vi "TestExecutive V3.vi"() -> ()   [LabVIEW 2025]
uses:
  controls/TestDefinition.ctl
  controls/SingleTest.ctl
  controls/TestType.ctl
  controls/Diode Test Options.ctl
  controls/HTR Test Options.ctl
  controls/TED4015 Status.ctl
  <vilib>/Utility/error.llb/DialogType.ctl
  <vilib>/addons/_JKI Toolkits/State Machine/_JKI_lib_State_Machine.llb/Select State(s)_err__jki_lib_state_machine.vi
  <vilib>/addons/_JKI Toolkits/State Machine/_JKI_lib_State_Machine.llb/Periodic Trigger__ogtk__JKI-SM__jki_lib_state_machine.vi
  subVIs/Globals.vi
panel:
  in  "Exit":bool
  out "Camera":string="HD Pro Webcam C920"
  out "TopFolderPath":path=path "D:/LTM Tests/November/Diode_check_25-11-13_18-53-57"
  out "TopFolderPrefix":string="Diode_check_25-11-13_18-53-57"
  out "Status":string="Waiting for Rising trigger. Target = -50.000000"
  in  "Main Tabs":T1(tab)=enum."Operating"
  in  "Cycles To Run":i32=1 min=1 max=200
  in  "Next1":bool
  in  "Loggers Directory":path=path "D:/LTM Tests/November"
  in  "Test Name":string="ChamberInstall_Pre-Test_Step47"
  in  "FFMPEG exe":path=path "C:/Program Files/FFMpeg/bin/ffmpeg.exe"
  in  "Path to Actuation Script":path=path "C:/Users/dpl/Documents/ob-egse/src/main.py"
  in  "StartCycle":i32
  in  "Tab Control":T2(tab)=enum."PSUs"
  in  "TVC_Temperatures":waveform(dbl)[](array[waveform])=[{"t0"=timestamp(3845904937.0241175 s since 1904-01-01), "dt"=1.0, "Y"=[-80.0], "attributes"=variant("NI_ChannelName"=variant(string "3A"))}, {"t0"=timestamp(3845904937.0241175 s since 1904-01-01), "dt"=1.0, "Y"=[0.1969585335155295], "attributes"=variant("NI_ChannelName"=variant(string "3B"))}, {"t0"=timestamp(3845904937.0241175 s since 1904-01-01), "dt"=1.0, "Y"=[0.2898606356704896], "attributes"=variant("NI_ChannelName"=variant(string "3C"))}, {"t0"=timestamp(3845904937.0241175 s since 1904-01-01), "dt"=1.0, "Y"=[0.3274623555028864], "attributes"=variant("NI_ChannelName"=variant(string "3D"))}, {"t0"=timestamp(3845904937.0241175 s since 1904-01-01), "dt"=1.0, "Y"=[0.3794250746071903], "attributes"=variant("NI_ChannelName"=variant(string "4A"))}, {"t0"=timestamp(3845904937.0241175 s since 1904-01-01), "dt"=1.0, "Y"=[0.7650917242886434], "attributes"=variant("NI_ChannelName"=variant(string "4B"))}, {"t0"=timestamp(3845904937.0241175 s since 1904-01-01), "dt"=1.0, "Y"=[0.4416685188806395], "attributes"=variant("NI_ChannelName"=variant(string "4C"))}, {"t0"=timestamp(3845904937.0241175 s since 1904-01-01), "dt"=1.0, "Y"=[0.7497510727682433], "attributes"=variant("NI_ChannelName"=variant(string "4D"))}, {"t0"=timestamp(3845904937.0241175 s since 1904-01-01), "dt"=1.0, "Y"=[0.8015992709050663], "attributes"=variant("NI_ChannelName"=variant(string "Target"))}]
  out "ChannelNames":string[](array[string])=["3A", "3B", "3C", "3D", "4A", "4B", "4C", "4D", "Target"]
  in  "ControlChannel":u16(ring) items=["3A", "3B", "3C", "3D", "4A", "4B", "4C", "4D", "Target"]
  in  "TLUP_Temperatures":waveform(dbl)[](array[waveform])=[{"t0"=timestamp(3820413812.102944 s since 1904-01-01), "dt"=1.0, "Y"=[23.56152], "attributes"=variant("NI_ChannelName"=variant(string "TLUP_0"))}, {"t0"=timestamp(3820413812.102944 s since 1904-01-01), "dt"=1.0, "Y"=[-999.0], "attributes"=variant("NI_ChannelName"=variant(string "TLUP_1"))}, {"t0"=timestamp(3820413812.102944 s since 1904-01-01), "dt"=1.0, "Y"=[-999.0], "attributes"=variant("NI_ChannelName"=variant(string "TLUP_2"))}, {"t0"=timestamp(3820413812.102944 s since 1904-01-01), "dt"=1.0, "Y"=[-999.0], "attributes"=variant("NI_ChannelName"=variant(string "TLUP_3"))}, {"t0"=timestamp(3820413812.102944 s since 1904-01-01), "dt"=1.0, "Y"=[nan], "attributes"=variant("NI_ChannelName"=variant(string "TLUP_4"))}, {"t0"=timestamp(3820413812.102944 s since 1904-01-01), "dt"=1.0, "Y"=[nan], "attributes"=variant("NI_ChannelName"=variant(string "TLUP_5"))}, {"t0"=timestamp(3820413812.102944 s since 1904-01-01), "dt"=1.0, "Y"=[nan], "attributes"=variant("NI_ChannelName"=variant(string "TLUP_6"))}, {"t0"=timestamp(3820413812.102944 s since 1904-01-01), "dt"=1.0, "Y"=[nan], "attributes"=variant("NI_ChannelName"=variant(string "TLUP_7"))}]
  in  "PSU_Monitor":waveform(dbl)[](array[waveform])=[{"t0"=timestamp(3845904937.0241175 s since 1904-01-01), "dt"=1.0, "Y"=[2.52], "attributes"=variant("NI_ChannelName"=variant(string "Board_Voltage_0"))}, {"t0"=timestamp(3845904937.0241175 s since 1904-01-01), "dt"=1.0, "Y"=[-0.009], "attributes"=variant("NI_ChannelName"=variant(string "Board_Voltage_0"))}, {"t0"=timestamp(3845904937.0241175 s since 1904-01-01), "dt"=1.0, "Y"=[-0.017], "attributes"=variant("NI_ChannelName"=variant(string "Board_Current_0"))}, {"t0"=timestamp(3845904937.0241175 s since 1904-01-01), "dt"=1.0, "Y"=[0.0], "attributes"=variant("NI_ChannelName"=variant(string "Board_Current_0"))}]
  in  "PSU Enable":bool
  in  "Heater Monitor":waveform(dbl)[](array[waveform])=[{"t0"=timestamp(3845904937.0241175 s since 1904-01-01), "dt"=1.0, "Y"=[-0.005], "attributes"=variant("NI_ChannelName"=variant(string "Heater_Voltage"))}, {"t0"=timestamp(3845904937.0241175 s since 1904-01-01), "dt"=1.0, "Y"=[-0.002], "attributes"=variant("NI_ChannelName"=variant(string "Heater_Current"))}]
  in  "Heater Enable":bool
  in  "COM Port":i32=21 min=1 max=63 step=1
  in  "Video Camera":u16(ring) items=["HD Pro Webcam C920"]
  in  "TED":waveform(dbl)[](graph)
  in  "TEC On":bool[](array[boolean])=[FALSE, FALSE]
  in  "TED Status":T3[](array[typedef])=[{"Output"=TRUE, "SetPoint"=0.0, "Temperature"=0.0, "Current"=0.5, "Voltage"=0.0, "CableTrip"=FALSE, "TransducerTrip"=FALSE, "OverTemp"=FALSE}, {"Output"=TRUE, "SetPoint"=0.0, "Temperature"=0.0, "Current"=0.5, "Voltage"=0.0, "CableTrip"=FALSE, "TransducerTrip"=FALSE, "OverTemp"=FALSE}]
  in  "LED_Stimulate":bool
  in  "LED_Illuminate":bool
  in  "Diode Currents":waveform(dbl)[](graph)=[{"t0"=timestamp(3845904936.8165374 s since 1904-01-01), "dt"=1.0, "Y"=[0.0]}, {"t0"=timestamp(3845904936.8165374 s since 1904-01-01), "dt"=1.0, "Y"=[0.0]}]
  in  "Next2":bool
  in  "Server IP":u16(ring) items=["localhost", "172.17.52.10"]
  in  "SaveTests":bool
  in  "TestDefinition":T4={"Test Sequence"=[{"TTrigger"=-130.0, "Direction"=enum."Falling", "TDelay"=0.0, "Type"=enum."No Test", "Pre-Log (s)"=0.0, "Duration (s)"=0.0, "Post-Log(s)"=0.0}, {"TTrigger"=-80.0, "Direction"=enum."Rising", "TDelay"=0.0, "Type"=enum."Heater Test", "Pre-Log (s)"=10.0, "Duration (s)"=15.0, "Post-Log(s)"=10.0}], "ActuationsPerLoop"=2, "Temperature Log Period(ms)"=1000, "PSU  Log Period (ms)"=1000, "Diode Test Options"={"Temp.Tol"=0.0, "Max IDark"=[], "Min ILight"=[], "Min TEC \nCurrent"=0.0, "Max TEC \nCurrent"=0.0}, "Heater Test Options"={"Heater Nominal Voltage (A)"=0.67, "Heater Voltage Tolerance (%)"=20.0}} {"Heater Test Options"."Heater Voltage Tolerance (%)" min=1.0 max=100.0; "Heater Test Options"."Heater Nominal Voltage (A)" min=0.0 max=1.0; "Test Sequence"."Post-Log(s)" format="%#_13g"; "Test Sequence"."Pre-Log (s)" format="%#_13g"; "Test Sequence"."Duration (s)" format="%#_13g"}
  in  "Next Button 3":bool
  in  "Tab Control 2":enum32{"Temperature", "Current/Voltages"}(tab)
  out "Temperatures":dynamicdata(graph)=[{"t0"=timestamp(3845904936.2041135 s since 1904-01-01), "dt"=1.0, "Y"=[-80.0], "attributes"=variant("NI_ChannelName"=variant(string "3A"))}, {"t0"=timestamp(3845904936.2041135 s since 1904-01-01), "dt"=1.0, "Y"=[0.1969585335155295], "attributes"=variant("NI_ChannelName"=variant(string "3B"))}, {"t0"=timestamp(3845904936.2041135 s since 1904-01-01), "dt"=1.0, "Y"=[0.2898606356704896], "attributes"=variant("NI_ChannelName"=variant(string "3C"))}, {"t0"=timestamp(3845904936.2041135 s since 1904-01-01), "dt"=1.0, "Y"=[0.3274623555028864], "attributes"=variant("NI_ChannelName"=variant(string "3D"))}, {"t0"=timestamp(3845904936.2041135 s since 1904-01-01), "dt"=1.0, "Y"=[0.3794250746071903], "attributes"=variant("NI_ChannelName"=variant(string "4A"))}, {"t0"=timestamp(3845904936.2041135 s since 1904-01-01), "dt"=1.0, "Y"=[0.7650917242886434], "attributes"=variant("NI_ChannelName"=variant(string "4B"))}, {"t0"=timestamp(3845904936.2041135 s since 1904-01-01), "dt"=1.0, "Y"=[0.4416685188806395], "attributes"=variant("NI_ChannelName"=variant(string "4C"))}, {"t0"=timestamp(3845904936.2041135 s since 1904-01-01), "dt"=1.0, "Y"=[0.7497510727682433], "attributes"=variant("NI_ChannelName"=variant(string "4D"))}, {"t0"=timestamp(3845904936.2041135 s since 1904-01-01), "dt"=1.0, "Y"=[0.8015992709050663], "attributes"=variant("NI_ChannelName"=variant(string "Target"))}, {"t0"=timestamp(3820413812.102944 s since 1904-01-01), "dt"=1.0, "Y"=[23.56152], "attributes"=variant("NI_ChannelName"=variant(string "TLUP_0"))}, {"t0"=timestamp(3820413812.102944 s since 1904-01-01), "dt"=1.0, "Y"=[-999.0], "attributes"=variant("NI_ChannelName"=variant(string "TLUP_1"))}, {"t0"=timestamp(3820413812.102944 s since 1904-01-01), "dt"=1.0, "Y"=[-999.0], "attributes"=variant("NI_ChannelName"=variant(string "TLUP_2"))}, {"t0"=timestamp(3820413812.102944 s since 1904-01-01), "dt"=1.0, "Y"=[-999.0], "attributes"=variant("NI_ChannelName"=variant(string "TLUP_3"))}, {"t0"=timestamp(3820413812.102944 s since 1904-01-01), "dt"=1.0, "Y"=[nan], "attributes"=variant("NI_ChannelName"=variant(string "TLUP_4"))}, {"t0"=timestamp(3820413812.102944 s since 1904-01-01), "dt"=1.0, "Y"=[nan], "attributes"=variant("NI_ChannelName"=variant(string "TLUP_5"))}, {"t0"=timestamp(3820413812.102944 s since 1904-01-01), "dt"=1.0, "Y"=[nan], "attributes"=variant("NI_ChannelName"=variant(string "TLUP_6"))}, {"t0"=timestamp(3820413812.102944 s since 1904-01-01), "dt"=1.0, "Y"=[nan], "attributes"=variant("NI_ChannelName"=variant(string "TLUP_7"))}]
  out "Current/Voltage":dynamicdata(graph)=[{"t0"=timestamp(3845904936.2041135 s since 1904-01-01), "dt"=1.0, "Y"=[-80.0], "attributes"=variant("NI_ChannelName"=variant(string "3A"))}, {"t0"=timestamp(3845904936.2041135 s since 1904-01-01), "dt"=1.0, "Y"=[0.1969585335155295], "attributes"=variant("NI_ChannelName"=variant(string "3B"))}, {"t0"=timestamp(3845904936.2041135 s since 1904-01-01), "dt"=1.0, "Y"=[0.2898606356704896], "attributes"=variant("NI_ChannelName"=variant(string "3C"))}, {"t0"=timestamp(3845904936.2041135 s since 1904-01-01), "dt"=1.0, "Y"=[0.3274623555028864], "attributes"=variant("NI_ChannelName"=variant(string "3D"))}, {"t0"=timestamp(3845904936.2041135 s since 1904-01-01), "dt"=1.0, "Y"=[0.3794250746071903], "attributes"=variant("NI_ChannelName"=variant(string "4A"))}, {"t0"=timestamp(3845904936.2041135 s since 1904-01-01), "dt"=1.0, "Y"=[0.7650917242886434], "attributes"=variant("NI_ChannelName"=variant(string "4B"))}, {"t0"=timestamp(3845904936.2041135 s since 1904-01-01), "dt"=1.0, "Y"=[0.4416685188806395], "attributes"=variant("NI_ChannelName"=variant(string "4C"))}, {"t0"=timestamp(3845904936.2041135 s since 1904-01-01), "dt"=1.0, "Y"=[0.7497510727682433], "attributes"=variant("NI_ChannelName"=variant(string "4D"))}, {"t0"=timestamp(3845904936.2041135 s since 1904-01-01), "dt"=1.0, "Y"=[0.8015992709050663], "attributes"=variant("NI_ChannelName"=variant(string "Target"))}, {"t0"=timestamp(3820413812.102944 s since 1904-01-01), "dt"=1.0, "Y"=[23.56152], "attributes"=variant("NI_ChannelName"=variant(string "TLUP_0"))}, {"t0"=timestamp(3820413812.102944 s since 1904-01-01), "dt"=1.0, "Y"=[-999.0], "attributes"=variant("NI_ChannelName"=variant(string "TLUP_1"))}, {"t0"=timestamp(3820413812.102944 s since 1904-01-01), "dt"=1.0, "Y"=[-999.0], "attributes"=variant("NI_ChannelName"=variant(string "TLUP_2"))}, {"t0"=timestamp(3820413812.102944 s since 1904-01-01), "dt"=1.0, "Y"=[-999.0], "attributes"=variant("NI_ChannelName"=variant(string "TLUP_3"))}, {"t0"=timestamp(3820413812.102944 s since 1904-01-01), "dt"=1.0, "Y"=[nan], "attributes"=variant("NI_ChannelName"=variant(string "TLUP_4"))}, {"t0"=timestamp(3820413812.102944 s since 1904-01-01), "dt"=1.0, "Y"=[nan], "attributes"=variant("NI_ChannelName"=variant(string "TLUP_5"))}, {"t0"=timestamp(3820413812.102944 s since 1904-01-01), "dt"=1.0, "Y"=[nan], "attributes"=variant("NI_ChannelName"=variant(string "TLUP_6"))}, {"t0"=timestamp(3820413812.102944 s since 1904-01-01), "dt"=1.0, "Y"=[nan], "attributes"=variant("NI_ChannelName"=variant(string "TLUP_7"))}]
  out "TEC Faults":bool[](array[boolean])
  out "Messages":string="13/11/2025 18:54:34: Diode Test Start\r\n13/11/2025 18:54:47: TEC Fault on TED-1\r\n13/11/2025 18:54:51: TEC Fault on TED-2\r\n13/11/2025 18:54:56: Low Light Current on Diode-1\r\n13/11/2025 18:54:56: Low Light Current on Diode-2\r\n13/11/2025 18:54:56: Low Light Current on Diode-1\r\n13/11/2025 18:54:56: Low Light Current on Diode-2\r\n13/11/2025 18:54:56: Low Light Current on Diode-1\r\n13/11/2025 18:54:56: Low Light Current on Diode-2\r\n13/11/2025 18:54:56: Low Light Current on Diode-1\r\n13/11/2025 18:54:56: Low Light Current on Diode-2\r\n13/11/2025 18:54:57: Low Light Current on Diode-1\r\n13/11/2025 18:54:57: Low Light Current on Diode-2\r\n13/11/2025 18:54:57: Low Light Current on Diode-1\r\n13/11/2025 18:54:57: Low Light Current on Diode-2\r\n13/11/2025 18:54:57: Low Light Current on Diode-1\r\n13/11/2025 18:54:57: Low Light Current on Diode-2\r\n13/11/2025 18:54:57: Low Light Current on Diode-1\r\n13/11/2025 18:54:57: Low Light Current on Diode-2\r\n13/11/2025 18:54:57: Low Light Current on Diode-1\r\n13/11/2025 18:54:57: Low Light Current on Diode-2\r\n13/11/2025 18:54:58: Low Light Current on Diode-1\r\n13/11/2025 18:54:58: Low Light Current on Diode-2\r\n13/11/2025 18:54:58: Low Light Current on Diode-1\r\n13/11/2025 18:54:58: Low Light Current on Diode-2\r\n13/11/2025 18:54:58: Low Light Current on Diode-1\r\n13/11/2025 18:54:58: Low Light Current on Diode-2\r\n13/11/2025 18:54:58: Low Light Current on Diode-1\r\n13/11/2025 18:54:58: Low Light Current on Diode-2\r\n13/11/2025 18:54:58: Low Light Current on Diode-1\r\n13/11/2025 18:54:58: Low Light Current on Diode-2\r\n13/11/2025 18:54:59: Low Light Current on Diode-1\r\n13/11/2025 18:54:59: Low Light Current on Diode-2\r\n13/11/2025 18:54:59: Low Light Current on Diode-1\r\n13/11/2025 18:54:59: Low Light Current on Diode-2\r\n13/11/2025 18:54:59: Low Light Current on Diode-1\r\n13/11/2025 18:54:59: Low Light Current on Diode-2\r\n13/11/2025 18:54:59: Low Light Current on Diode-1\r\n13/11/2025 18:54:59: Low Light Current on Diode-2\r\n13/11/2025 18:54:59: Low Light Current on Diode-1\r\n13/11/2025 18:54:59: Low Light Current on Diode-2\r\n13/11/2025 18:55:00: Low Light Current on Diode-1\r\n13/11/2025 18:55:00: Low Light Current on Diode-2\r\n13/11/2025 18:55:00: Low Light Current on Diode-1\r\n13/11/2025 18:55:00: Low Light Current on Diode-2\r\n13/11/2025 18:55:00: Low Light Current on Diode-1\r\n13/11/2025 18:55:00: Low Light Current on Diode-2\r\n13/11/2025 18:55:00: Low Light Current on Diode-1\r\n13/11/2025 18:55:00: Low Light Current on Diode-2\r\n13/11/2025 18:55:00: Low Light Current on Diode-1\r\n13/11/2025 18:55:00: Low Light Current on Diode-2\r\n13/11/2025 18:55:01: Low Light Current on Diode-1\r\n13/11/2025 18:55:01: Low Light Current on Diode-2\r\n13/11/2025 18:55:01: Low Light Current on Diode-1\r\n13/11/2025 18:55:01: Low Light Current on Diode-2\r\n"
  out "ACT Fault":bool
  out "TVC_StopAfterCycle":bool
  out "Diode Logging":bool
  out "Master Logging":bool=TRUE
  out "DelayRemaining":string
  out "HTR On":bool
  out "Trigger Point Reading":dbl=-80.0
  out "ACT Logging":bool
  out "HTR Log":bool
  out "TVC_CyclesRemaining":i32=1
  in  "TVC_CycleNumber":i32
  out "HTR_Fault":bool
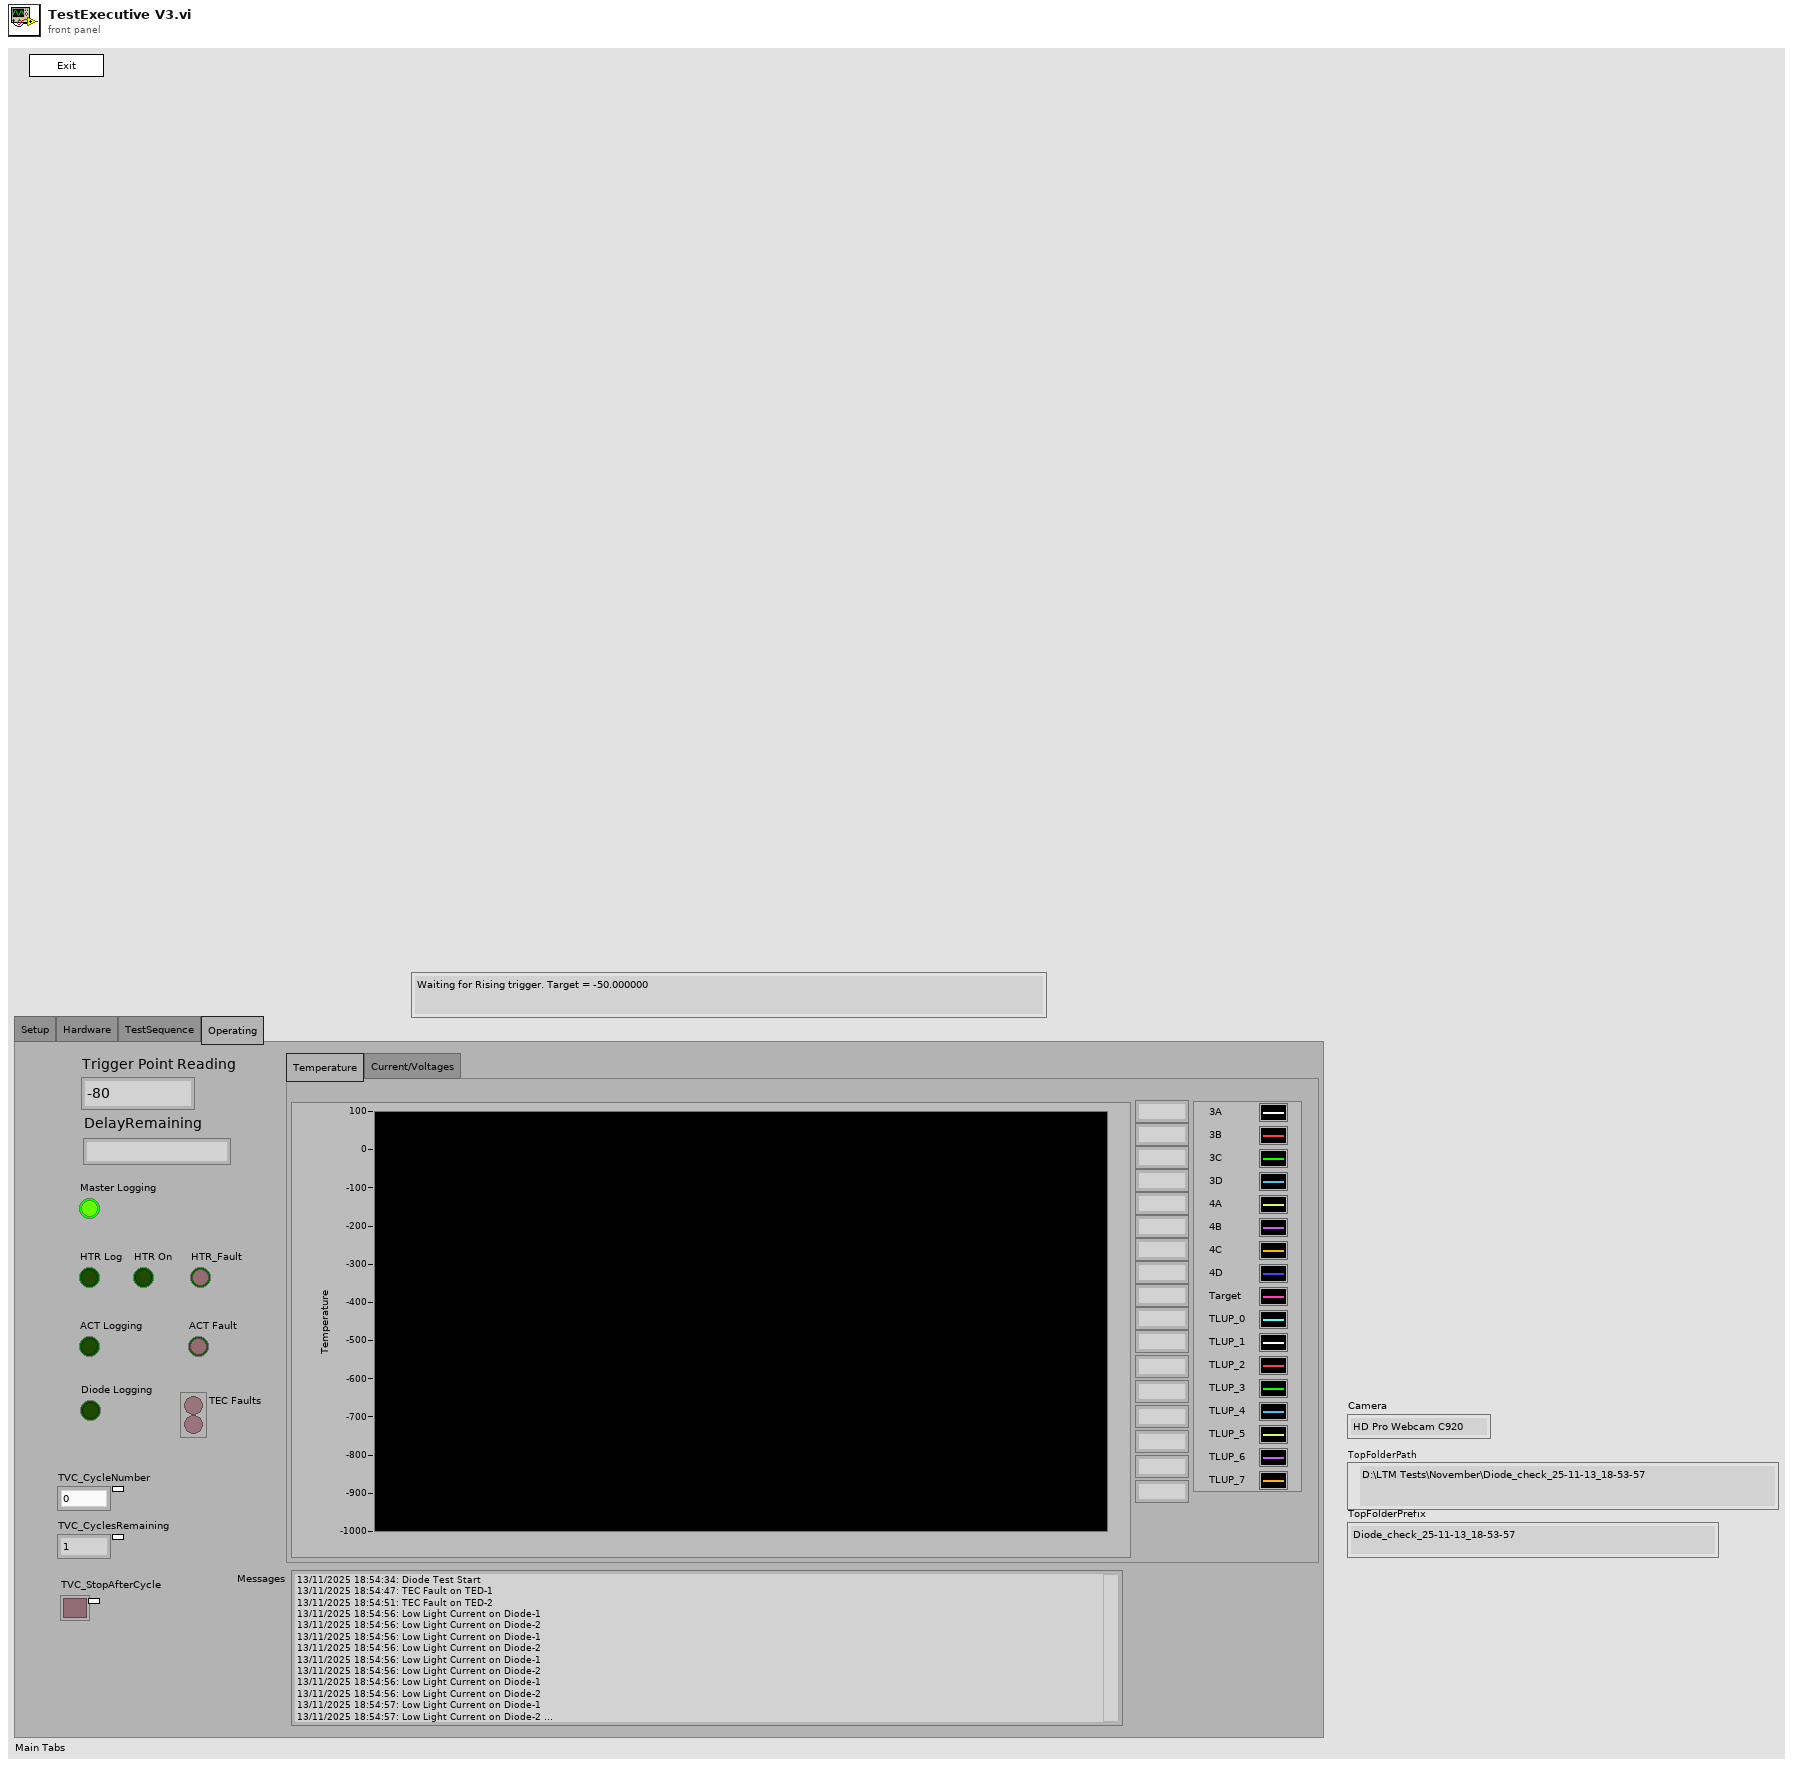
[diagram p1: front panel]
types:
  T1 = enum32{"Setup", "Hardware", "TestSequence", "Operating"}
  T2 = enum32{"Temperatures", "PSUs", "TED4015s", "Diodes"}
  T3 = typedef "TED4015 Status.ctl" = cluster{"Output":bool, "SetPoint":dbl, "Temperature":dbl, "Current":dbl, "Voltage":dbl, "CableTrip":bool, "TransducerTrip":bool, "OverTemp":bool}
  T4 = typedef "TestDefinition.ctl" = cluster{"Test Sequence":T5[], "ActuationsPerLoop":i32, "Temperature Log Period(ms)":i64, "PSU  Log Period (ms)":i64, "Diode Test Options":T7, "Heater Test Options":T8}
  T5 = typedef "SingleTest.ctl" = cluster{"TTrigger":dbl, "Direction":enum16{"Rising", "Falling"}, "TDelay":dbl, "Type":T6, "Pre-Log (s)":dbl, "Duration (s)":dbl, "Post-Log(s)":dbl}
  T6 = typedef "TestType.ctl" = enum16{"No Test", "Heater Test", "Actuation Test", "Diode Test"}
  T7 = typedef "Diode Test Options.ctl" = cluster{"Temp.Tol":dbl, "Max IDark":dbl[], "Min ILight":dbl[], "Min TEC \nCurrent":dbl, "Max TEC \nCurrent":dbl}
  T8 = typedef "HTR Test Options.ctl" = cluster{"Heater Nominal Voltage (A)":dbl, "Heater Voltage Tolerance (%)":dbl}
  T9 = enum32{"Invalid", "Standard", "Closed", "Hidden", "Minimized", "Maximized"}
  T10 = enum32{"invalid app kind", "Development System", "Run Time System", "Student Edition", "Embedded LabVIEW", "Evaluation", "Custom"}
  T11 = enum32{"Invalid Status", "Unconnected", "Active", "Idle", "Error", "Connecting"}
  T12 = cluster{"Core":cluster{"Current VI Reference":refnum<vi>, "Close Panel on Exit?":bool}, "CurrentCycle":i32, "TestNumber":i32, "TopFolderPath":path, "LogFilePath":path, "TestPrefix":string, "CurrentTest":T5, "TestDefinitions":T4}
  T13 = typedef "DialogType.ctl" = u16
  T14 = cluster{"Current VI Reference":refnum<vi>, "Close Panel on Exit?":bool}
  T15 = typedef "LVDataSocketStatusTypeDef.ctl" = cluster{"Code":enum32{"Invalid Status", "Unconnected", "Active", "Idle", "Error", "Connecting"}, "Text":string}
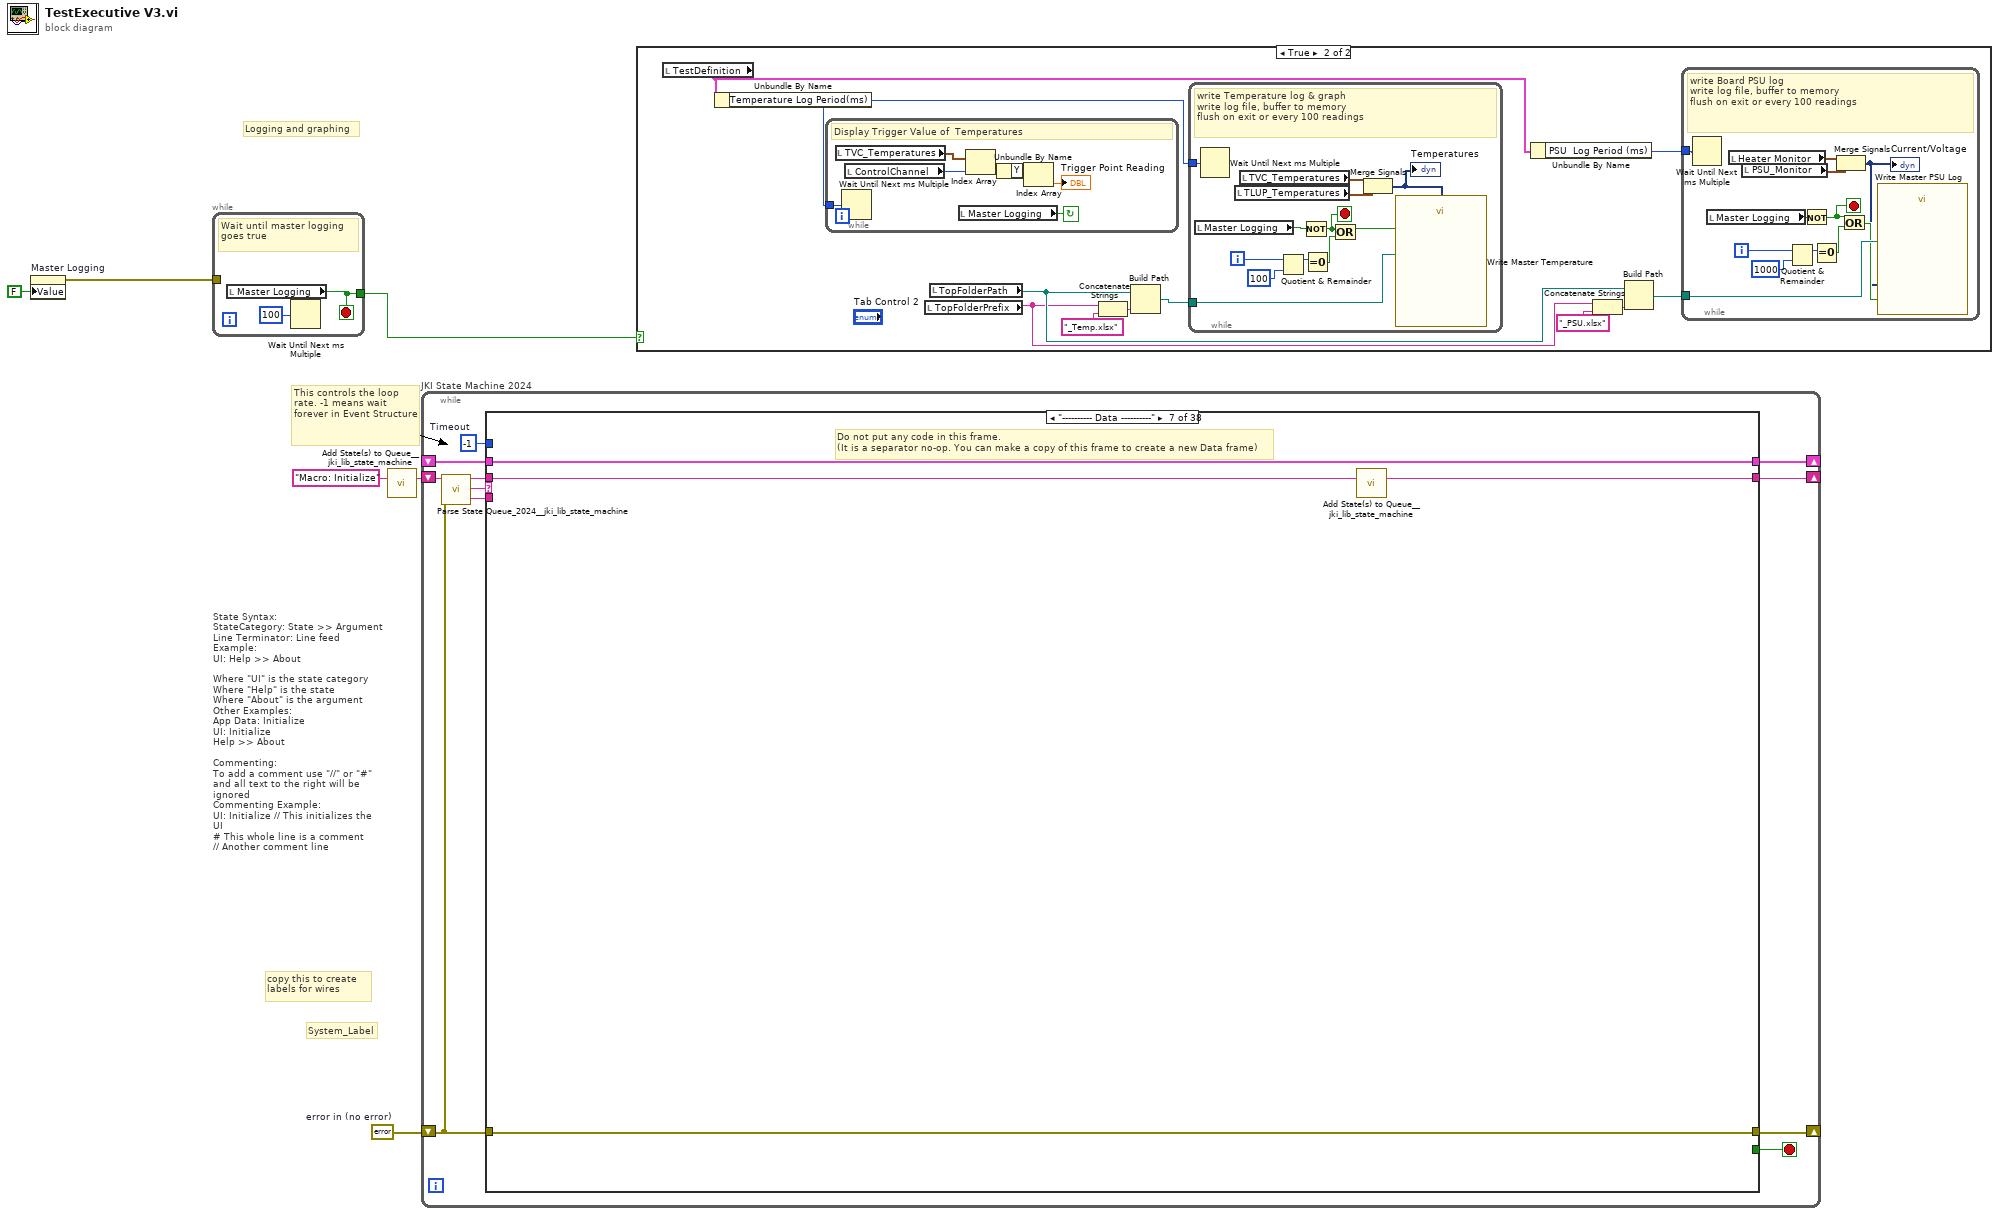
[diagram p0: block diagram]
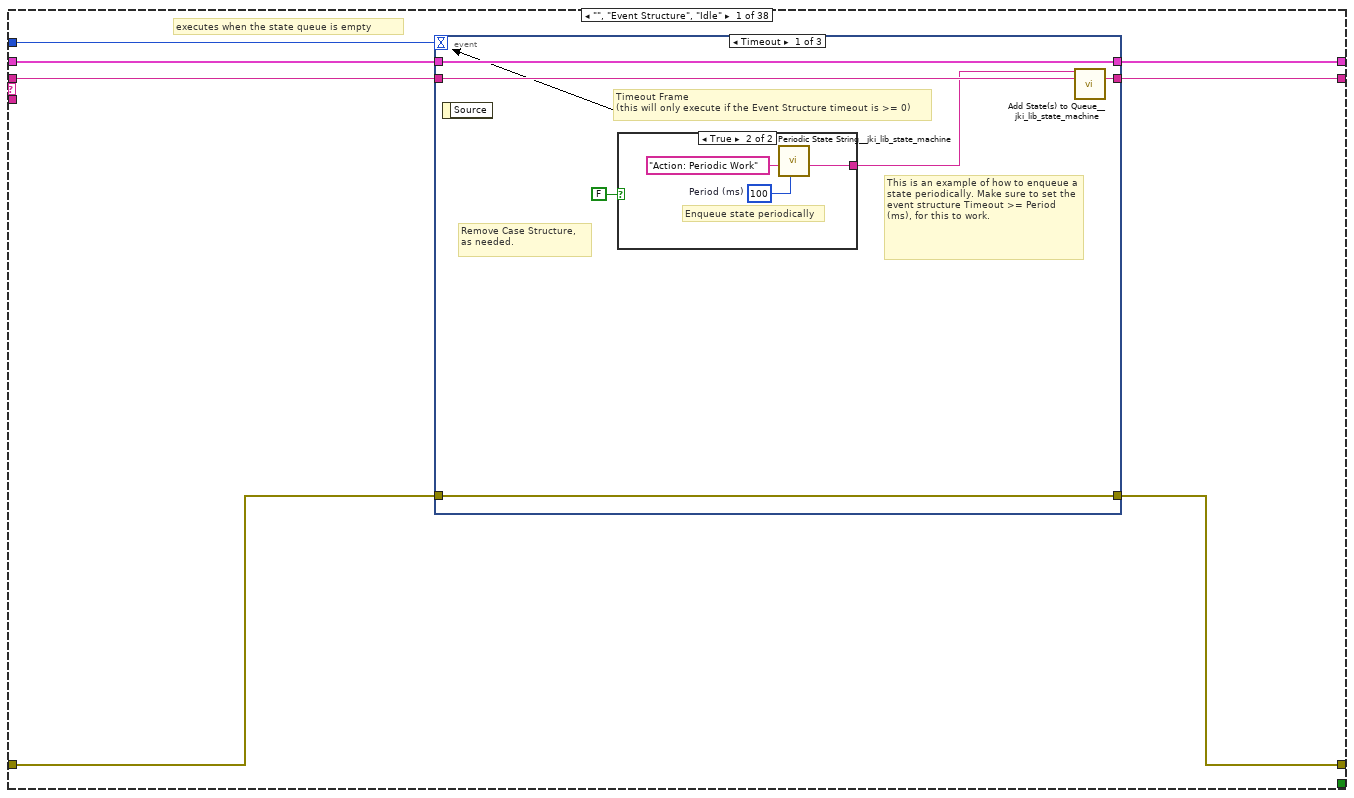
[diagram p2: hidden frame]
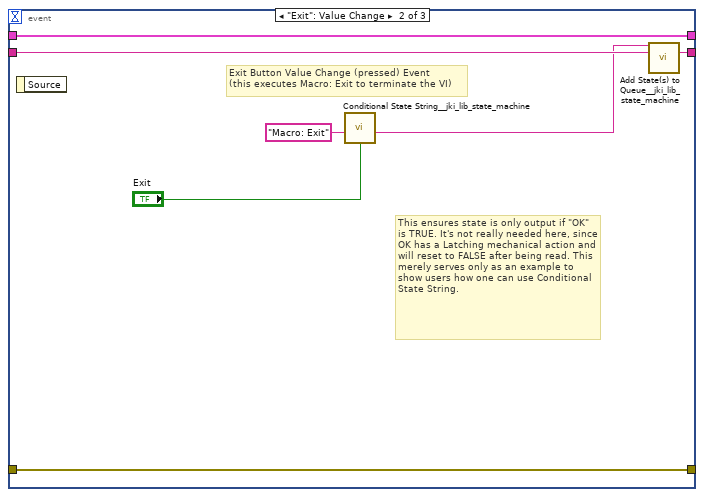
[diagram p4: hidden frame]
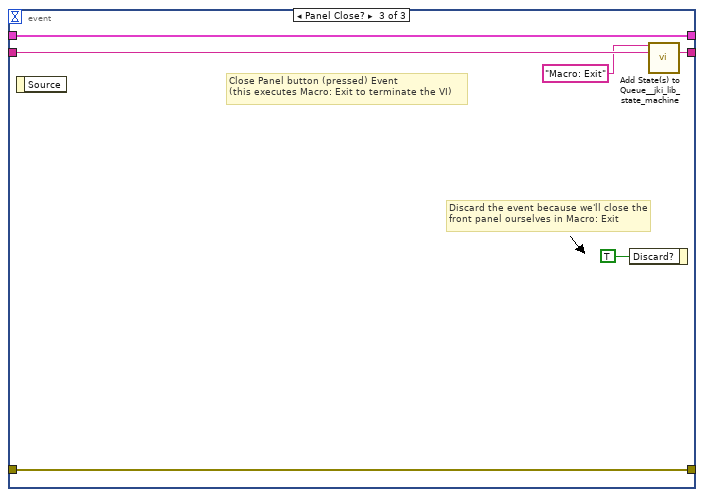
[diagram p5: hidden frame]
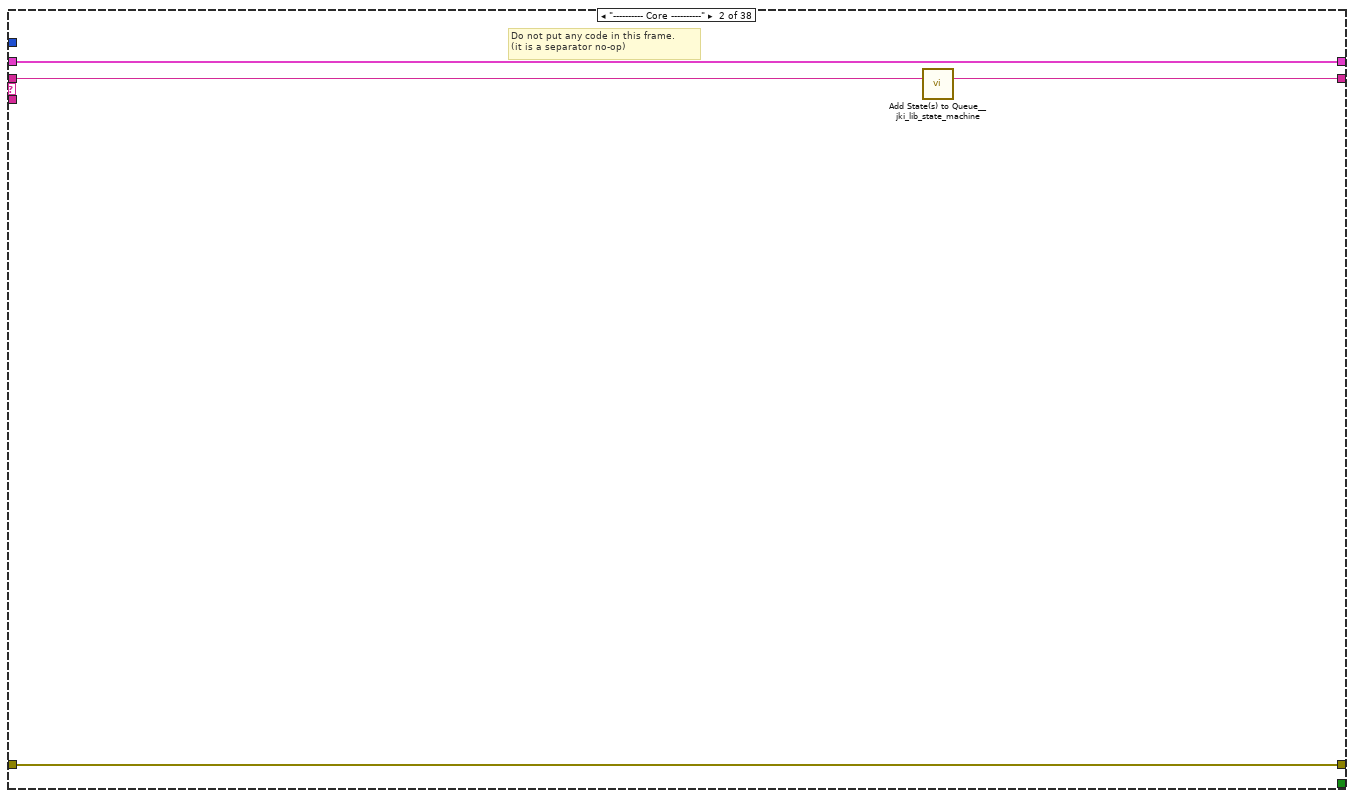
[diagram p6: hidden frame]
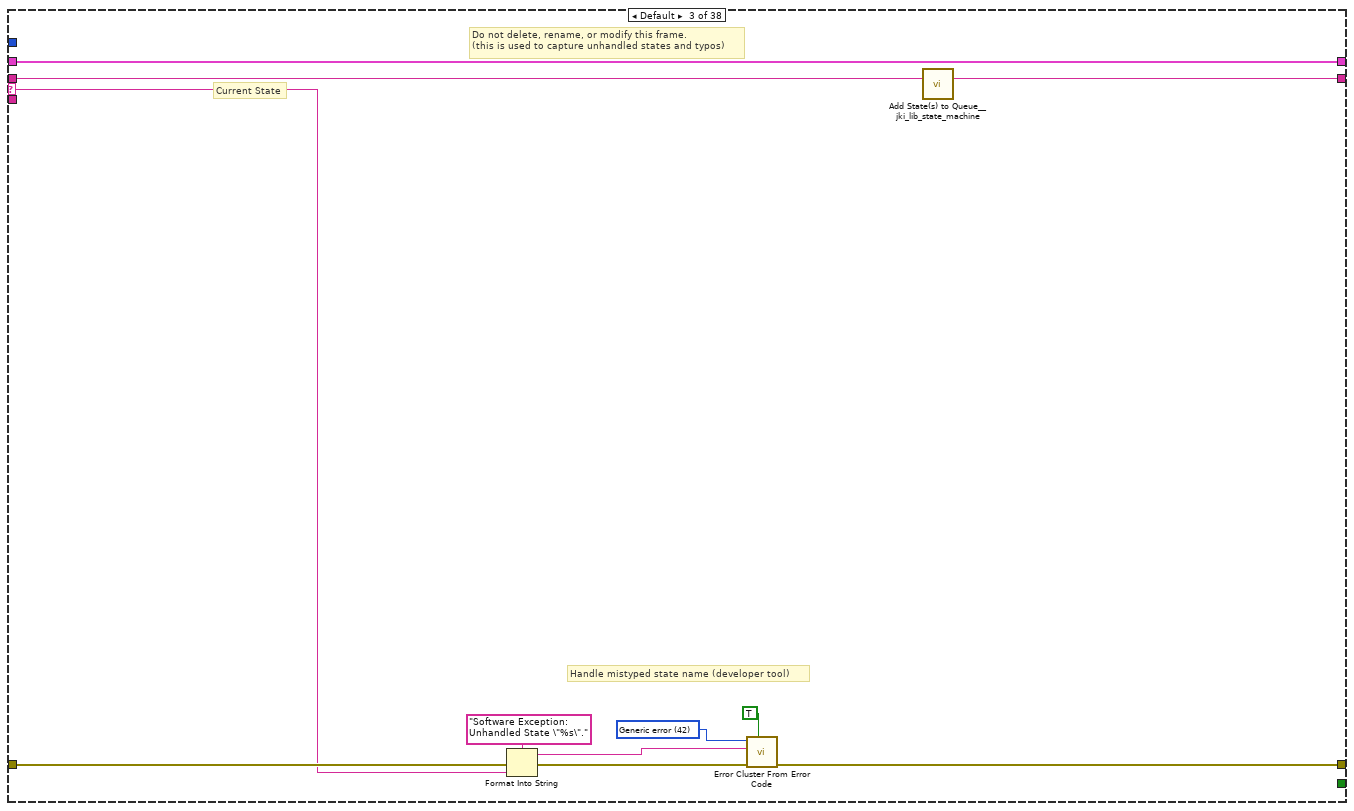
[diagram p7: hidden frame]
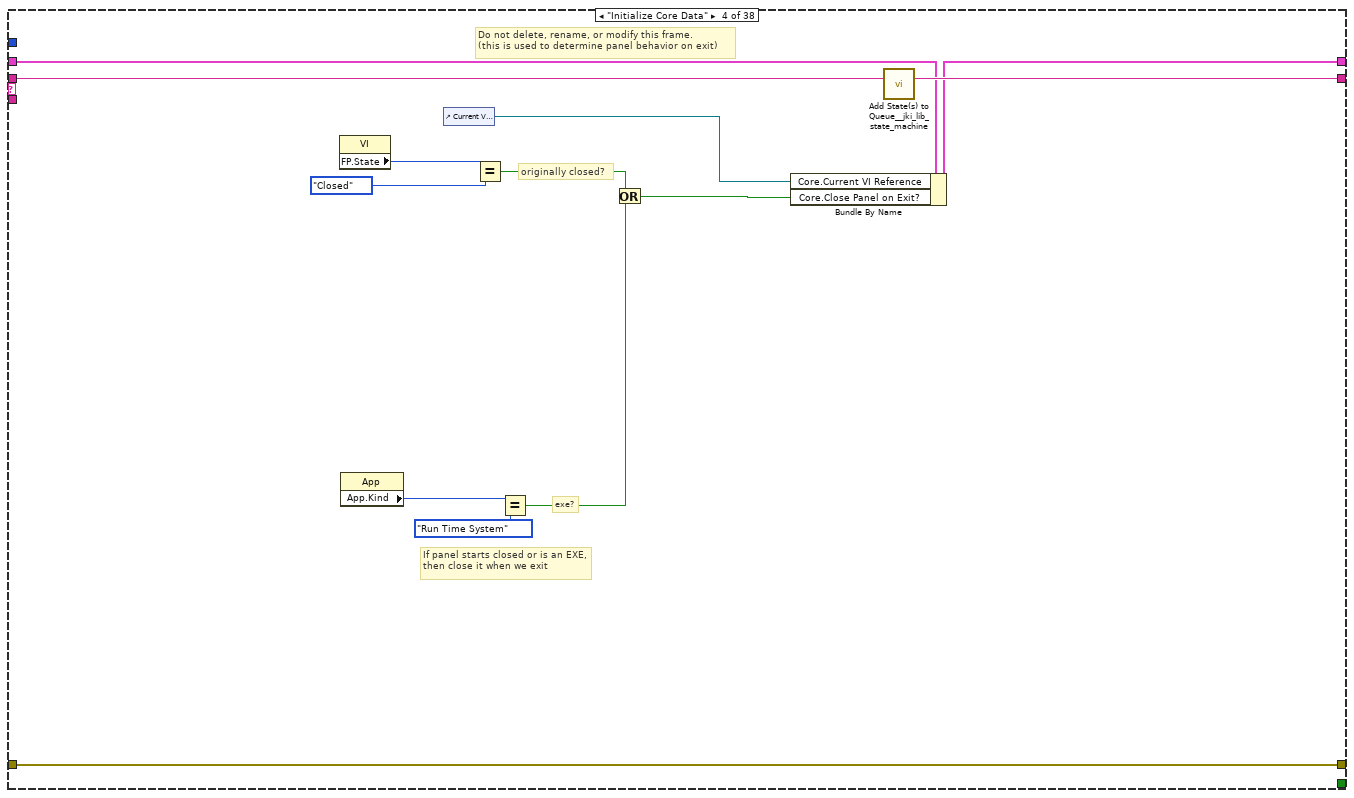
[diagram p8: hidden frame]
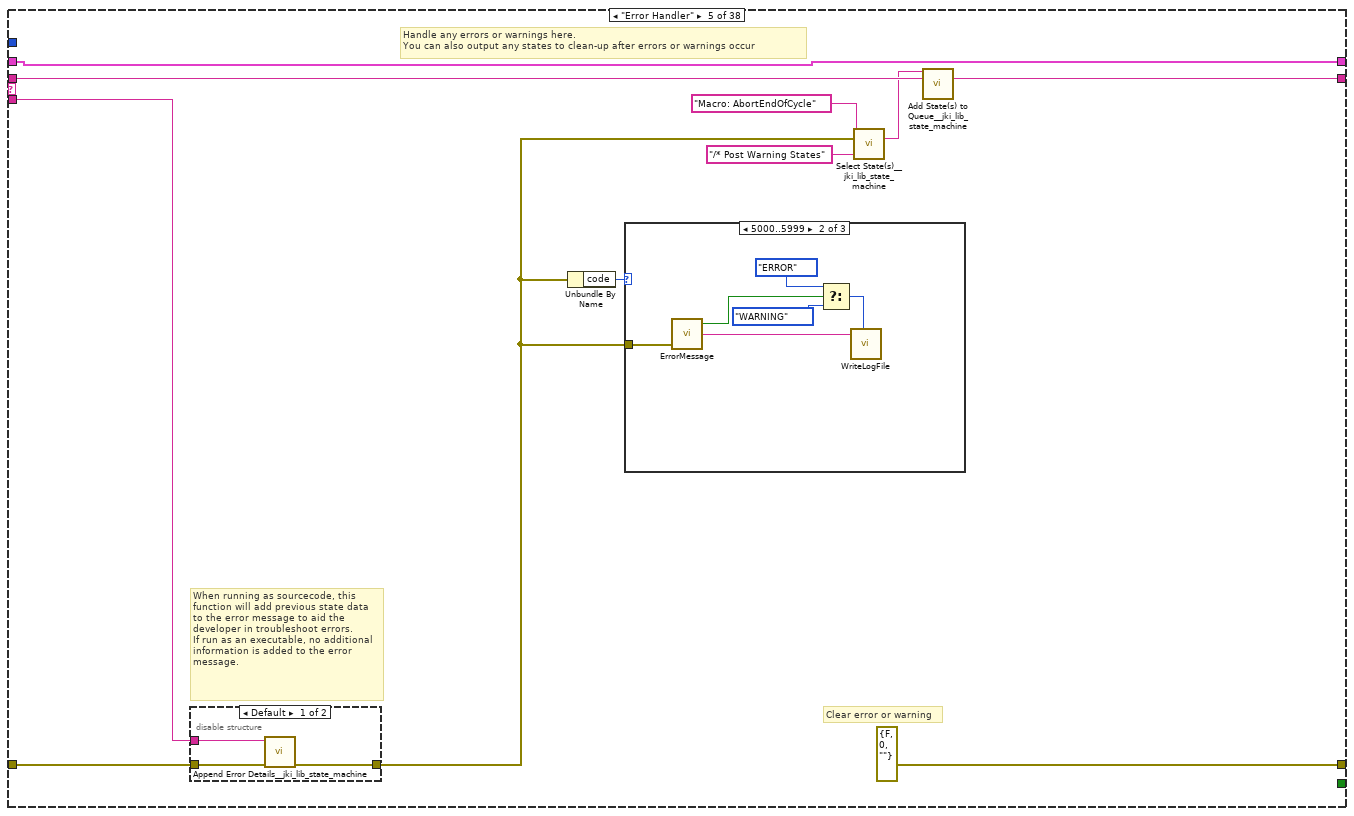
[diagram p9: hidden frame]
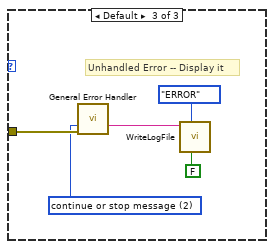
[diagram p11: hidden frame]
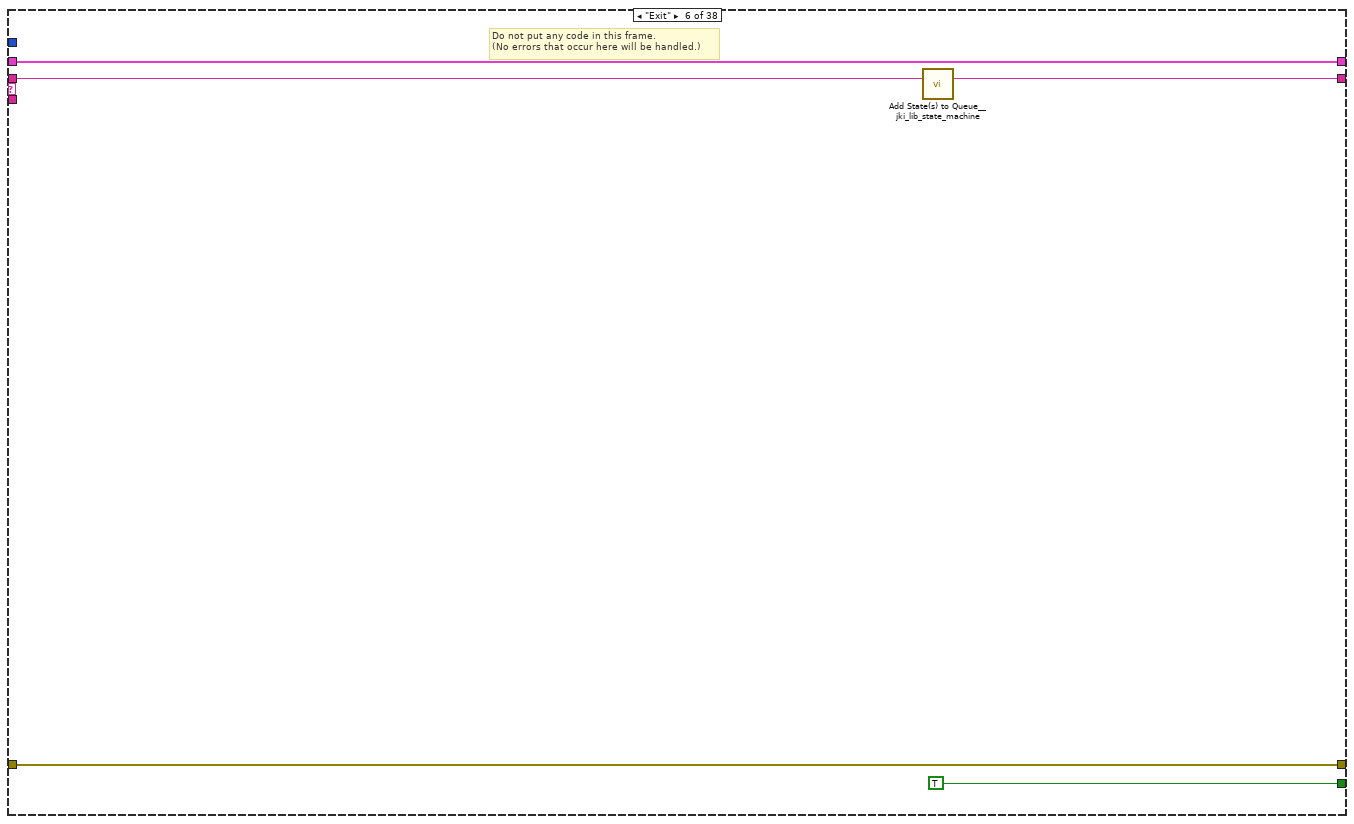
[diagram p13: hidden frame]
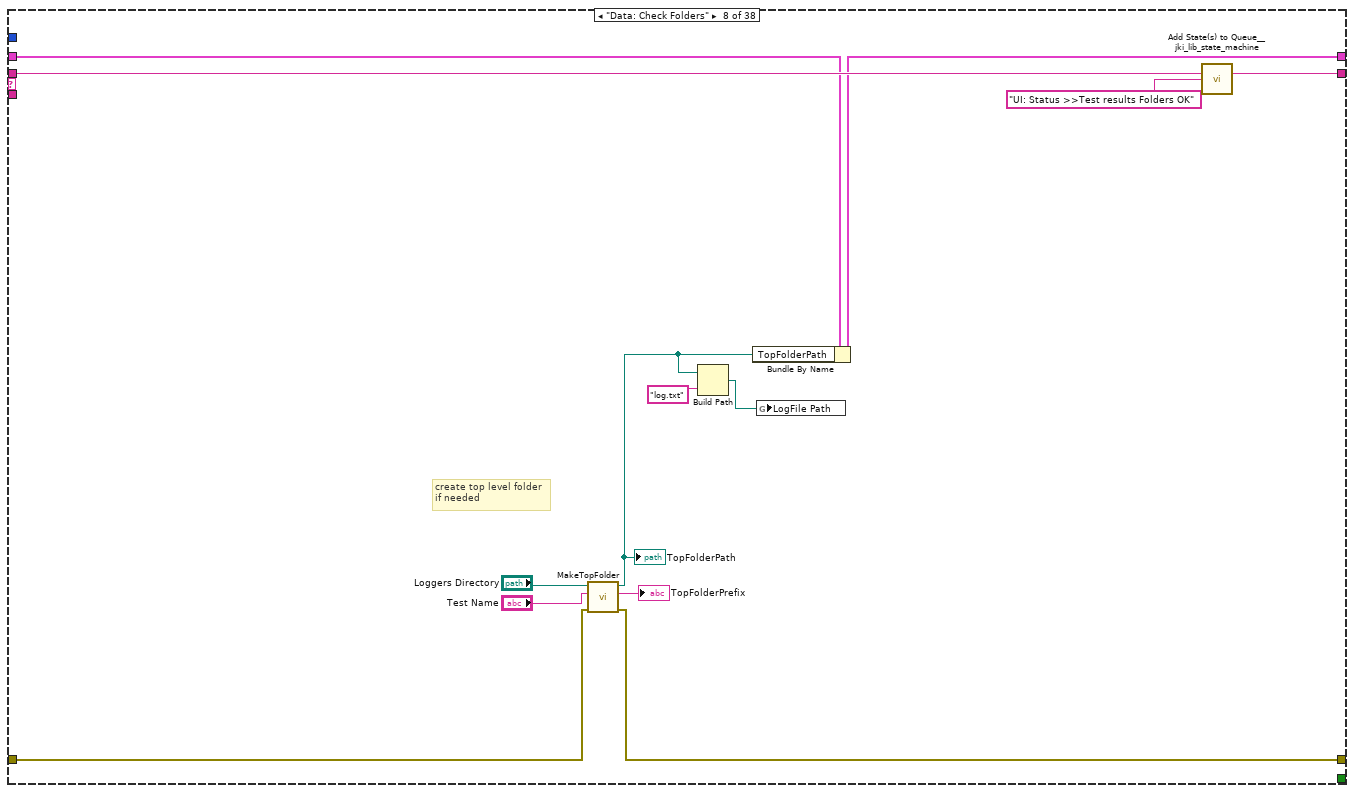
[diagram p14: hidden frame]
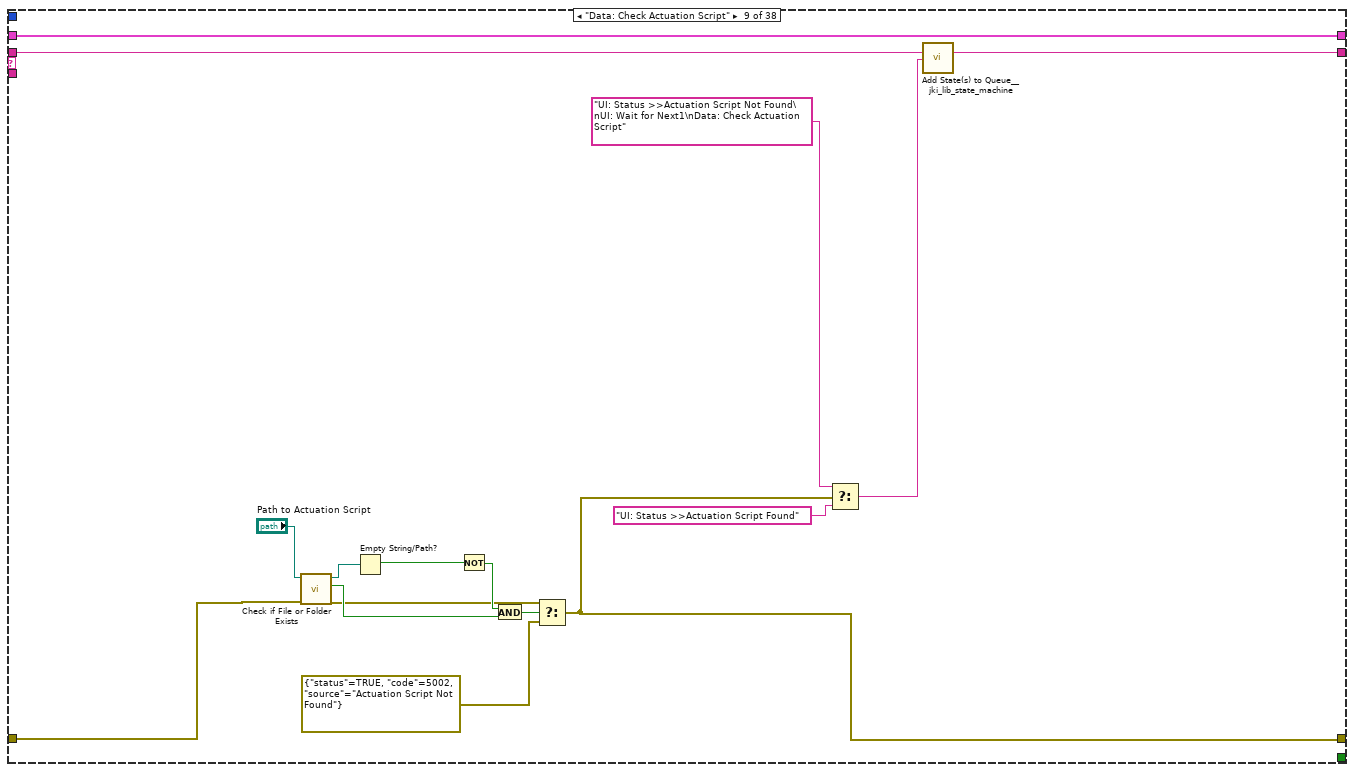
[diagram p15: hidden frame]
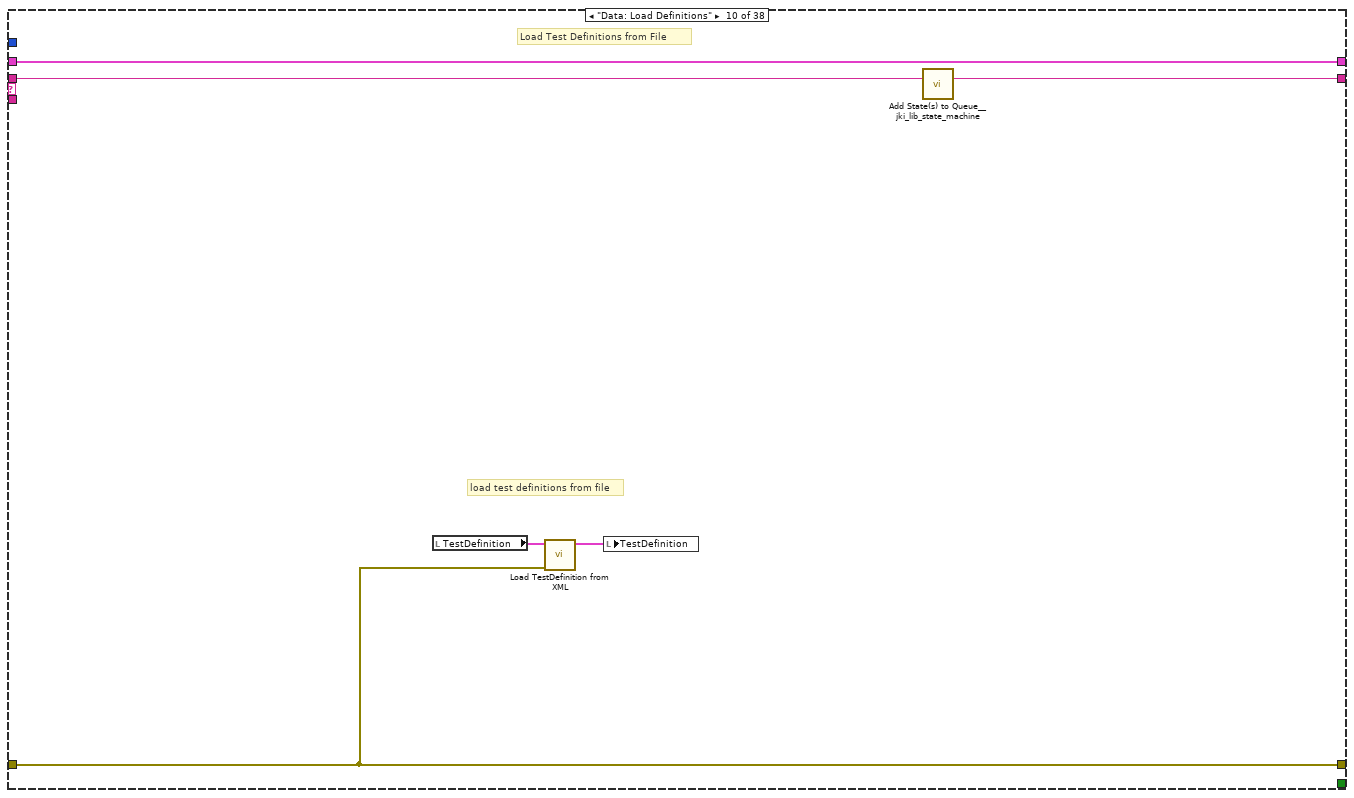
[diagram p16: hidden frame]
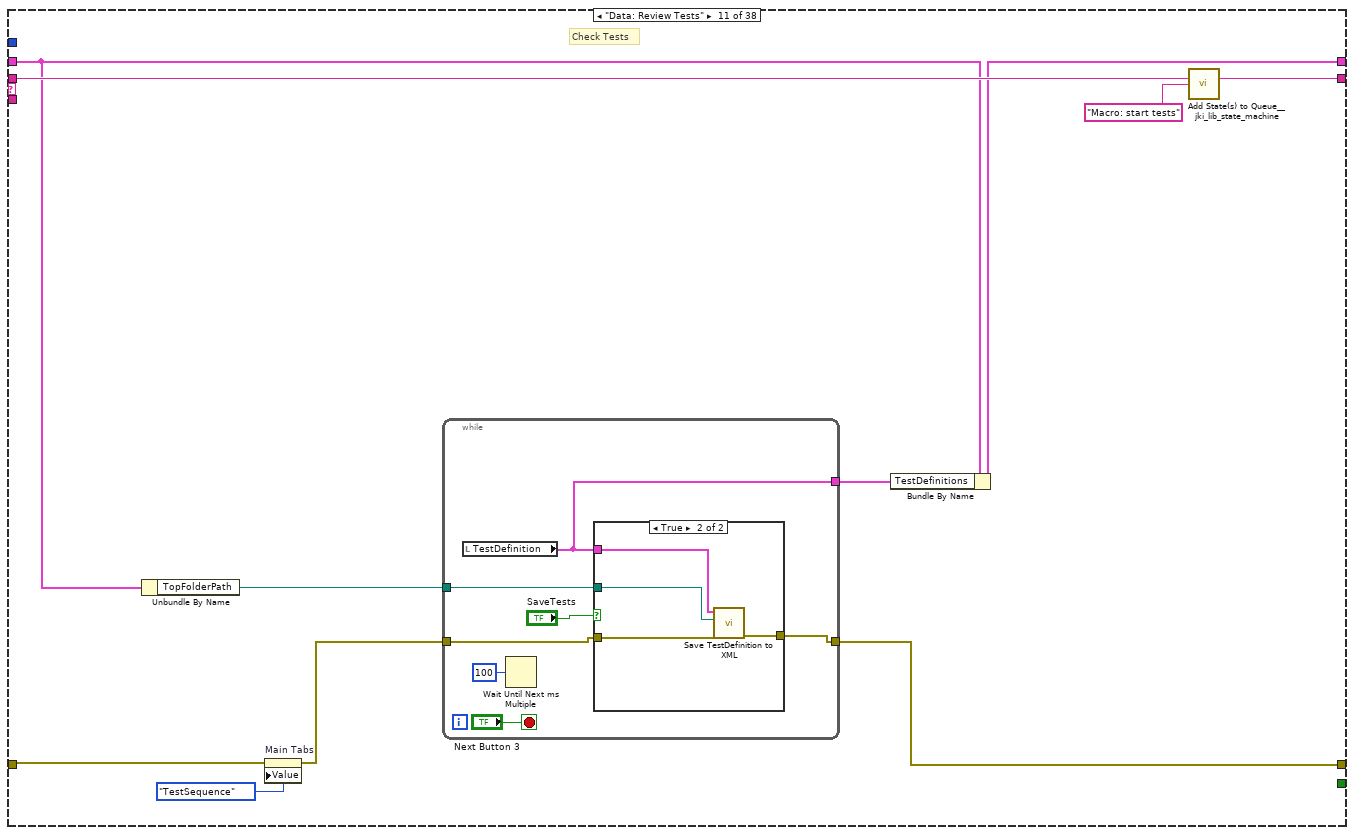
[diagram p17: hidden frame]
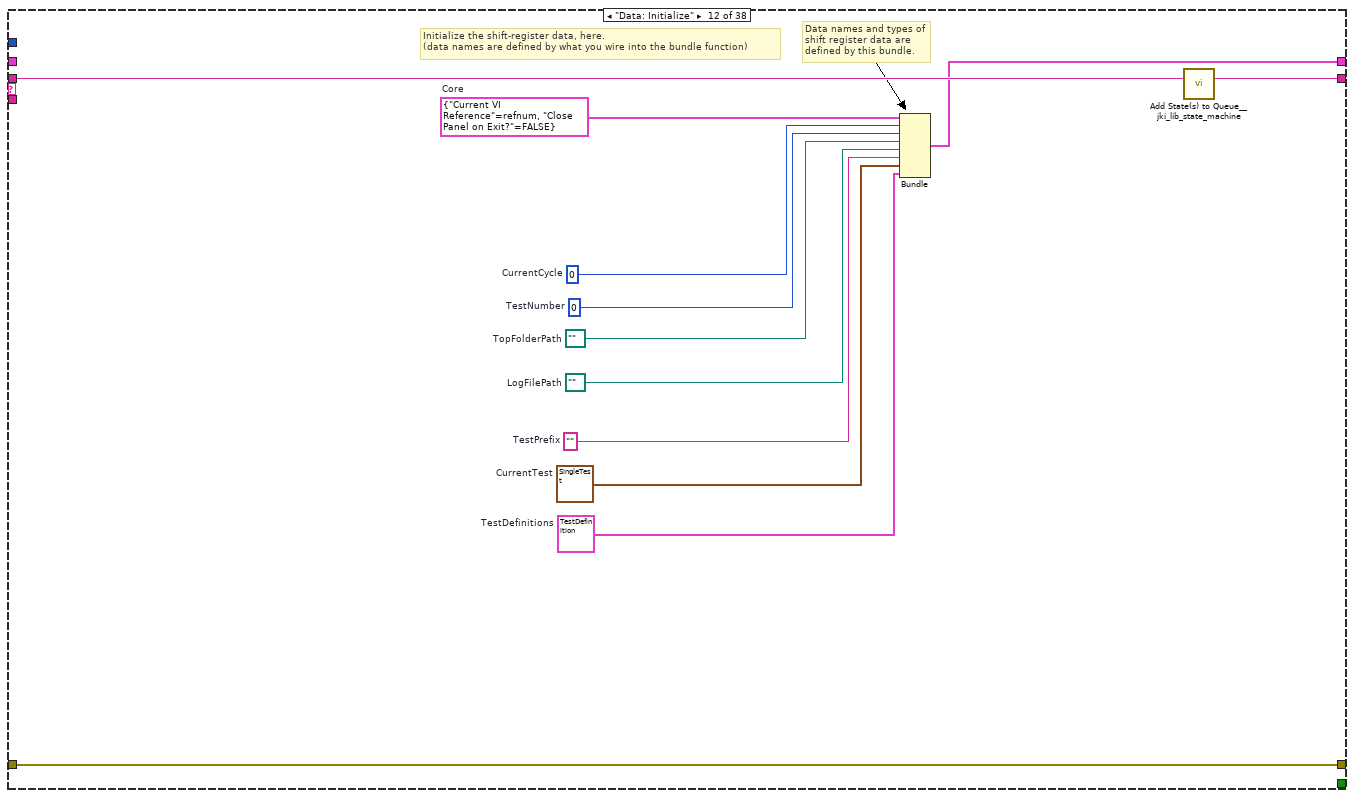
[diagram p19: hidden frame]
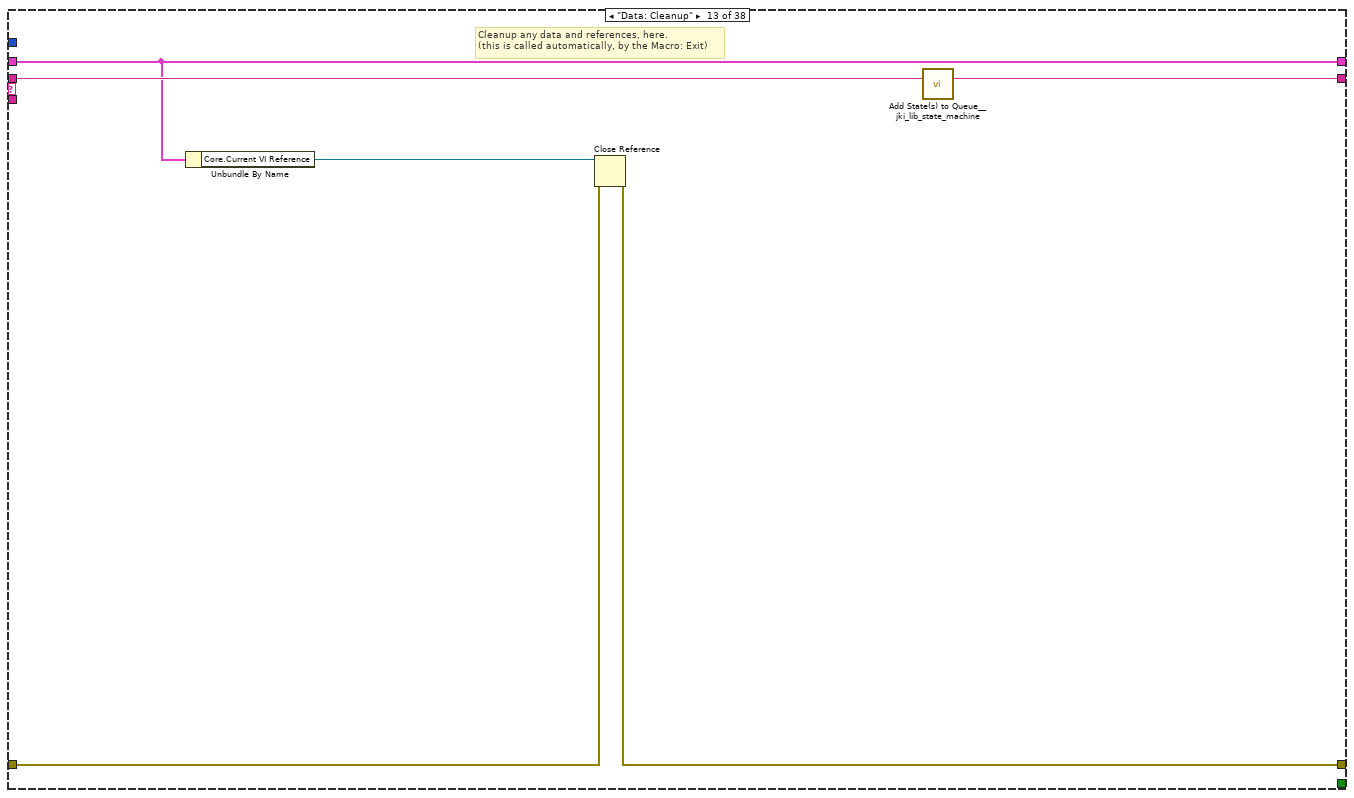
[diagram p20: hidden frame]
diagram:
  w1 = errorcluster {"status"=FALSE, "code"=0, "source"=""}  # error in (no error)
  # "State Syntax:\nStateCategory: State >> Argument\nLine Terminator: Line feed\nExample:\nUI: Help >> About\n\nWhere \"UI\" is the state category\nWhere \"Help\" is the state\nWhere \"About\" is the argument\nOther Examples:\nApp Data: Initialize\nUI: Initialize\nHelp >> About\n\nCommenting:\nTo add a comment use \"//\" or \"#\" and all text to the right will be ignored\nCommenting Example:\nUI: Initialize // This initializes the UI\n# This whole line is a comment\n// Another comment line"
  # "copy this to create labels for wires"
  # "This controls the loop rate. -1 means wait forever in Event Structure"
  # "System_Label"
  # "Logging and graphing"
  n1 = property on="Master Logging" class="Bool (strict)"("Value"=FALSE ("Master Logging")) -> (error out=w6:errorcluster)  [unwired: 2 in, 1 out]
  n2 = while {
    tunnel: [w7] -> w4
    tunnel: w6 -> [_]
    stop <- w7 stop-if-true
    # "Wait until master logging goes true"
    n3 = local read "Master Logging"() -> (w7:bool)
    n4 = Wait Until Next ms Multiple(millisecond multiple=u32 100) -> ()  [unwired: 1 out]
  }
  n5 = call <vilib>:"Add State(s) to Queue__jki_lib_state_machine.vi"("State(s) in (\"\")"="Macro: Initialize") -> ("States Out"=w3:string)  [unwired: 14 in]
  n6 = while "JKI State Machine 2024" {
    shift-right: [w12] -> _
    shift-left: _ -> [w11]
    shift-right: [w15] -> _
    shift-left: w1 -> [w9]
    shift-right: [w14] -> _
    shift-left: w3 -> [w16]
    stop <- w13 stop-if-true
    w10 = -1  # Timeout
    n7 = call <vilib>:"Parse State Queue_2024__jki_lib_state_machine.vi"("State Queue"=w16, "Error In (no error)"=w9) -> ("Remaining States"=w18:string, "Current State"=w19:string, "Arguments"=w17:string)  [unwired: 11 in]
    n8 = case shown="\"---------- Data ----------\"" w19 {
      selector: w19 -> [_ _ w53 _ _ _ _ _ _ _ _ _ _ _ _ _ _ _ _ _ _ _ _ _ _ _ _ _ _ _ _ _ _ _ _ _ _ _]
      tunnel: w18 -> [w26 w52 w57 w76 w87 w107 w111 w124 w140 w146 w157 w181 w187 w191 w195 w207 w214 w220 w239 w257 w268 w337 w342 w355 w372 w384 w440 w478 w488 w565 w584 w673 w689 w698 w702 w711 w736 w745]
      tunnel: w17 -> [_ _ _ _ w83 _ _ _ _ _ _ _ _ _ _ _ _ w215 _ w252 w262 _ _ w347 _ _ _ _ _ _ _ _ _ _ _ _ _ _]
      tunnel: w11 -> [w24 w49 w55 w69 w77 w105 w108 w122 w138 w144 w148 _ w182 w188 w192 w205 w212 w218 w237 w255 w264 w334 w339 w353 w370 w374 w438 w476 w484 w549 w580 w667 w685 w696 w699 w709 w734 w743]
      tunnel: [w23 w50 w59 w73 errorcluster {"status"=FALSE, "code"=0, "source"=""} ("error out") w104 w109 w117 w128 w141 w153 w178 w183 w189 w193 w204 w208 w216 w224 w253 w265 w335 w340 w348 w358 w381 w428 w473 w483 w539 w578 w668 w686 w693 w700 w703 w725 w738] -> w15
      tunnel: w9 -> [w20 w50 w58 w73 w84 w104 w109 w118 w130 w141 w155 w178 w184 w189 w193 w204 w209 w217 w225 w254 w266 w335 w340 w344 w365 w382 w428 w472 w482 w561 w579 w669 w687 w693 w700 w704 w728 w742]
      tunnel: [w25 w51 w56 w75 w86 w106 w110 w123 w139 w145 w156 w180 w186 w190 w194 w206 w213 w219 w238 w256 w267 w336 w341 w354 w371 w383 w439 w477 w487 w564 w583 w672 w688 w697 w701 w710 w735 w744] -> w14
      tunnel: [_ _ _ _ _ TRUE _ _ _ _ _ _ _ _ _ _ _ _ _ _ _ _ _ _ _ _ _ _ _ _ _ _ _ _ _ _ _ _] -> w13
      tunnel: [w22 w49 w55 w74 w77 w105 w108 w115 w138 w144 w150 w179 w182 w188 w192 w205 w212 w218 w237 w255 w264 w334 w339 w353 w364 w373 w434 w475 w486 w563 w582 w671 w685 w696 w699 w709 w734 w743] -> w12
      tunnel: w10 -> [w21 _ _ _ _ _ _ _ _ _ _ _ _ _ _ _ _ _ _ _ _ _ _ _ _ _ _ _ _ _ _ _ _ _ _ _ _ _]
      frame "", "Event Structure", "Idle" {
        # "executes when the state queue is empty"
        n9 = event shown="[0] Timeout" {
          selector: _ -> [_ _ _]
          dyn-events: _ -> [_ _ _]
          timeout: w21 -> [_ _ _]
          tunnel: w26 -> [w32 w42 w48]
          tunnel: [w31 w41 w47] -> w25
          tunnel: w24 -> [w29 w39 w45]
          tunnel: [w30 w40 w46] -> w23
          tunnel: w20 -> [w30 w40 w46]
          tunnel: [w29 w39 w45] -> w22
          event Timeout {
            # "Remove Case Structure, as needed."
            # "This is an example of how to enqueue a state periodically. Make sure to set the event structure Timeout >= Period (ms), for this to work."
            # "Timeout Frame\n(this will only execute if the Event Structure timeout is >= 0)"
            n10 = event-data() -> ()  [unwired: 1 in, 1 out]
            n11 = case shown="True" FALSE {
              tunnel: [_ w35] -> w28
              frame False {
              }
              frame True {
                w33 = u32 100  # Period (ms)
                # "Enqueue state periodically"
                n12 = call <vilib>:"Periodic State String__jki_lib_state_machine.vi"("Period (ms)"=w33, "State"="Action: Periodic Work") -> ("State Out"=w35:string)  [unwired: 9 in]
              }
            }
            n13 = call <vilib>:"Add State(s) to Queue__jki_lib_state_machine.vi"("State(s) in Front (\"\")"=w28, "State(s) in (\"\")"=w32) -> ("States Out"=w31:string)  [unwired: 13 in]
          }
          event "Exit": Value Change {
            # "This ensures state is only output if \"OK\" is TRUE. It's not really needed here, since OK has a Latching mechanical action and will reset to FALSE after being read. This merely serves only as an example to show users how one can use Conditional State String."
            # "Exit Button Value Change (pressed) Event\n(this executes Macro: Exit to terminate the VI)"
            n14 = event-data() -> ()  [unwired: 1 in, 1 out]
            n15 = call <vilib>:"Conditional State String__jki_lib_state_machine.vi"("Do State(s)?"="Exit", "State"="Macro: Exit") -> ("State Out"=w36:string)  [unwired: 7 in]
            n16 = call <vilib>:"Add State(s) to Queue__jki_lib_state_machine.vi"("State(s) in Front (\"\")"=w36, "State(s) in (\"\")"=w42) -> ("States Out"=w41:string)  [unwired: 13 in]
          }
          event Panel Close? {
            # "Discard the event because we'll close the front panel ourselves in Macro: Exit"
            # "Close Panel button (pressed) Event\n(this executes Macro: Exit to terminate the VI)"
            n17 = event-data() -> ()  [unwired: 1 in, 1 out]
            n18 = event-data("Discard?"=TRUE) -> ()  [unwired: 1 in, 1 out]
            n19 = call <vilib>:"Add State(s) to Queue__jki_lib_state_machine.vi"("State(s) in Front (\"\")"="Macro: Exit", "State(s) in (\"\")"=w48) -> ("States Out"=w47:string)  [unwired: 13 in]
          }
        }
      }
      frame "---------- Core ----------" {
        # "Do not put any code in this frame.\n(it is a separator no-op)"
        n20 = call <vilib>:"Add State(s) to Queue__jki_lib_state_machine.vi"("State(s) in (\"\")"=w52) -> ("States Out"=w51:string)  [unwired: 14 in]
      }
      frame Default {
        w62 = 42 items=["No error", "Argument error", "Memory is full", "Out of zone", "End of file", "File already open", "Generic file I/O error", "File not found", "File permission error", "Disk is full", "Duplicate path", "Too many files open", "System feature not enabled", "Resource file not found", "Cannot add resource", "Resource not found", "Image not found", "Image memory error", "Pen does not exist", "Config type invalid", "Config token not found", "Config parse error", "Config memory error", "Bad external code format", "Bad external code offset", "External code not present", "Null window", "Destroy window error", "Null menu", "Print aborted", "Bad print record", "Print driver error", "Windows error during printing", "Memory error during printing", "Print dialog error", "Generic print error", "Invalid device refnum", "Device not found", "Device parameter error", "Device unit error", "Cannot open device", "Device call aborted", "Generic error", "Cancelled by user", "Object ID too low", "Object ID too high", "Object not in heap", "Unknown heap", "Unknown object (invalid DefProc)", "Unknown object (DefProc not in table)", "Message out of range", "Invalid (null) method", "Unknown message", "Manager call not supported", "Bad address", "Network operation in progress", "Network operation timed out", "Connection is busy", "Network attribute not supported", "Network error", "Address in use", "System out of memory", "Connection aborted", "Connection refused", "Not connected", "Already connected", "Connection closed", "Initialization error (interapplication manager)", "Bad occurrence", "Wait on unbound occurrence handler", "Occurrence queue overflow", "Datalog type conflict", "Unused", "Unrecognized type (interapplication manager)", "Memory corrupt", "Failed to make temporary DLL", "Old CIN version", "Drag socket not found", "Failed to load drop-object", "Failed to register OLE object", "Failed to release OLE object", "Format specifier type mismatch", "Unknown format specifier", "Too few format specifiers", "Too many format specifiers", "Scan failed", "Newer CIN version", "Error converting to variant", "Runtime menu error", "Password tampered", "Variant attribute not found", "Incompatible variant data type", "Event data is not available", "Event Store is not present", "Occurrence is not found", "Event Queue is not created", "Event info is not available", "Refnum passed is NULL", "Error retrieving Class GUID", "Error retrieving CoClass GUID", "Error retrieving TypeLib GUID.", "Bad built application magic bytes.", "Specific driver is different from the specific driver associated with the Logical Name.", "There is no session opened to the class driver.", "Max Error", "MAX - Error with config objects", "MAX - Error loading configuration", "MAX - Group not supported"]
        # "Current State"
        # "Do not delete, rename, or modify this frame.\n(this is used to capture unhandled states and typos)"
        # "Handle mistyped state name (developer tool)"
        n21 = Format Into String(format string="Software Exception: Unhandled State \"%s\"." ("message"), error in=w58, w53) -> (resulting string=w61:string, error out=w60:errorcluster)  [unwired: 1 in]
        n22 = call <vilib>:"Error Cluster From Error Code.vi"("show call chain? (False)"=TRUE, "error in (no error)"=w60, "error message (\"\")"=w61, "error code (0)"=w62) -> ("error out"=w59:errorcluster)  [unwired: 5 in]
        n23 = call <vilib>:"Add State(s) to Queue__jki_lib_state_machine.vi"("State(s) in (\"\")"=w57) -> ("States Out"=w56:string)  [unwired: 14 in]
      }
      frame "Initialize Core Data" {
        # "Do not delete, rename, or modify this frame.\n(this is used to determine panel behavior on exit)"
        # "originally closed?"
        # "exe?"
        # "If panel starts closed or is an EXE, then close it when we exit"
        n24 = property class="VI"() -> ("FP.State"=w66:T9)  [unwired: 2 in, 2 out]
        n25 = property class="App"() -> ("App.Kind"=w72:T10)  [unwired: 2 in, 2 out]
        n26 = control-ref of="Current VI Reference"() -> (w67:refnum<vi>)
        n27 = Equal?(x=w66, y=T9."Closed" ("Front Panel Window:State")) -> (x = y?=w64:bool)
        n28 = Equal?(x=w72, y=T10."Run Time System" ("Application:Kind")) -> (x = y?=w70:bool)
        n29 = Or(x=w64, y=w70) -> (x .or. y?=w68:bool)
        n30 = Bundle By Name(cluster=w69, "Core.Current VI Reference"=w67, "Core.Close Panel on Exit?"=w68) -> (w74:T12)
        n31 = call <vilib>:"Add State(s) to Queue__jki_lib_state_machine.vi"("State(s) in (\"\")"=w76) -> ("States Out"=w75:string)  [unwired: 14 in]
      }
      frame "Error Handler" {
        # "When running as sourcecode, this function will add previous state data to the error message to aid the developer in troubleshoot errors.\nIf run as an executable, no additional information is added to the error message."
        # "Handle any errors or warnings here.\nYou can also output any states to clean-up after errors or warnings occur"
        # "Clear error or warning"
        n32 = disable-structure shown="Default" {
          disable-tunnel: w84 -> [w101 w102]
          disable-tunnel: w83 -> [w100 _]
          disable-tunnel: [w99 w102] -> w78
          frame condition #0 (active) {
            n33 = call <vilib>:"Append Error Details__jki_lib_state_machine.vi"("error in (no error)"=w101, "Previous State and Argument(s)"=w100) -> ("error out"=w99:errorcluster)  [unwired: 9 in]
          }
          frame condition #1 {
          }
        }
        n34 = Unbundle By Name(w78) -> ("code"=w79:i32)
        n35 = case shown="5000..5999" w79 {
          tunnel: w78 -> [_ w93 w98]
          frame 0 {
          }
          frame 5000..5999 {
            n36 = call "ErrorMessage.vi"("error in (no error)"=w93) -> ("Message String"=w92:string, "error?"=w88:bool)  [unwired: 3 in]
            n37 = Select(t=enum16{"INFO", "WARNING", "ERROR"}."ERROR" ("Type"), s=w88, f=enum16{"INFO", "WARNING", "ERROR"}."WARNING") -> (s? t:f=w90:enum16{"INFO", "WARNING", "ERROR"})
            n38 = call "WriteLogFile.vi"("Type"=w90, "Message"=w92) -> ()  [unwired: 9 in, 1 out]
          }
          frame Default {
            w94 = T13 2 items=["no dialog", "OK message", "continue or stop message", "OK message + warnings", "continue/stop + warnings"] ("type of dialog (OK msg:1)")
            # "Unhandled Error -- Display it"
            n39 = call <vilib>:"General Error Handler.vi"("type of dialog (OK msg:1)"=w94, "error in (no error)"=w98) -> ("message"=w96:string)  [unwired: 9 in, 4 out]
            n40 = call "WriteLogFile.vi"("Prepend TimeStamp"=FALSE, "Type"=enum16{"INFO", "WARNING", "ERROR"}."ERROR", "Message"=w96) -> ()  [unwired: 8 in, 1 out]
          }
        }
        n41 = call-poly <vilib>:"Select State(s)__jki_lib_state_machine.vi"("State(s) if True (\"\")"="Macro: AbortEndOfCycle", "Select"=w78, "State(s) if False (\"\")"="/* Post Warning States") -> ("States Out"=w81:string)  [unwired: 12 in]
        n42 = call <vilib>:"Add State(s) to Queue__jki_lib_state_machine.vi"("State(s) in Front (\"\")"=w81, "State(s) in (\"\")"=w87) -> ("States Out"=w86:string)  [unwired: 13 in]
      }
      frame "Exit" {
        # "Do not put any code in this frame.\n(No errors that occur here will be handled.)"
        n43 = call <vilib>:"Add State(s) to Queue__jki_lib_state_machine.vi"("State(s) in (\"\")"=w107) -> ("States Out"=w106:string)  [unwired: 14 in]
      }
      frame "---------- Data ----------" {
        # "Do not put any code in this frame.\n(It is a separator no-op. You can make a copy of this frame to create a new Data frame)"
        n44 = call <vilib>:"Add State(s) to Queue__jki_lib_state_machine.vi"("State(s) in (\"\")"=w111) -> ("States Out"=w110:string)  [unwired: 14 in]
      }
      frame "Data: Check Folders" {
        # "create top level folder\nif needed"
        n45 = call "MakeTopFolder.vi"("error in (no error)"=w118, "Comment"="Test Name", "Loggers"="Loggers Directory") -> ("error out"=w117:errorcluster, "TopFolderPrefix"=→"TopFolderPrefix":string, "TestFolderPath"=w114:path)  [unwired: 6 in]
        "TopFolderPath" <- w114
        n46 = Build Path(base path=w114, name or relative path="log.txt") -> (appended path=w112:path)
        n47 = Bundle By Name(cluster=w122, "TopFolderPath"=w114) -> (w115:T12)
        n48 = global write "Globals.vi" "LogFile Path"(w112) -> ()
        n49 = call <vilib>:"Add State(s) to Queue__jki_lib_state_machine.vi"("State(s) in (\"\")"=w124, "State(s) at Back (\"\")"="UI: Status >>Test results Folders OK" ("State(s) at Back (\"\")")) -> ("States Out"=w123:string)  [unwired: 13 in]
      }
      frame "Data: Check Actuation Script" {
        n50 = call <vilib>:"Check if File or Folder Exists.vi"("error in (no error)"=w130, "path"="Path to Actuation Script") -> ("error out"=w132:errorcluster, "file or folder exists?"=w137:bool, "dup path"=w133:path)  [unwired: 7 in]
        n51 = Empty String/Path?(string/path=w133) -> (empty?=w135:bool)
        n52 = Not(x=w135) -> (.not. x?=w136:bool)
        n53 = And(x=w136, y=w137) -> (x .and. y?=w134:bool)
        n54 = Select(t=w132, s=w134, f=errorcluster {"status"=TRUE, "code"=5002, "source"="Actuation Script Not Found"} ("error constant")) -> (s? t:f=w128:errorcluster)
        n55 = Select(t="UI: Status >>Actuation Script Not Found\nUI: Wait for Next1\nData: Check Actuation Script" ("State(s) at Back (\"\")"), s=w128, f="UI: Status >>Actuation Script Found" ("State(s) at Back (\"\")")) -> (s? t:f=w125:string)
        n56 = call <vilib>:"Add State(s) to Queue__jki_lib_state_machine.vi"("State(s) in (\"\")"=w140, "State(s) at Back (\"\")"=w125) -> ("States Out"=w139:string)  [unwired: 13 in]
      }
      frame "Data: Load Definitions" {
        # "load test definitions from file"
        # "Load Test Definitions from File"
        n57 = local read "TestDefinition"() -> (w142:T4)
        n58 = call "Load TestDefinition from XML.vi"("error in (no error)"=w141, "TestDefinition"=w142) -> ("User Specified Out"=w143:T4)  [unwired: 8 in, 1 out]
        n59 = local write "TestDefinition"(w143) -> ()
        n60 = call <vilib>:"Add State(s) to Queue__jki_lib_state_machine.vi"("State(s) in (\"\")"=w146) -> ("States Out"=w145:string)  [unwired: 14 in]
      }
      frame "Data: Review Tests" {
        # "Check Tests"
        n61 = Unbundle By Name(w148) -> ("TopFolderPath"=w147:path)
        n62 = property on="Main Tabs" class="TabCtl (strict)"(error in=w155, "Value"=T1."TestSequence" ("Main Tabs")) -> (error out=w154:errorcluster)  [unwired: 1 in, 1 out]
        n63 = while {
          tunnel: w154 -> [w161]
          tunnel: [w160] -> w153
          tunnel: [w159] -> w149
          tunnel: w147 -> [w158]
          stop <- "Next Button 3" stop-if-true
          n64 = local read "TestDefinition"() -> (w159:T4)
          n65 = Wait Until Next ms Multiple(millisecond multiple=u32 100) -> ()  [unwired: 1 out]
          n66 = case shown="True" "SaveTests" {
            tunnel: [w165 w169] -> w160
            tunnel: w161 -> [w165 w168]
            tunnel: w159 -> [_ w167]
            tunnel: w158 -> [_ w166]
            frame False {
            }
            frame True {
              n67 = call "Save TestDefinition to XML.vi"("error in (no error)"=w168, "SaveDir"=w166, "TestDefinition"=w167) -> ("error out"=w169:errorcluster)  [unwired: 8 in]
            }
          }
        }
        n68 = Bundle By Name(cluster=w148, "TestDefinitions"=w149) -> (w150:T12)
        n69 = call <vilib>:"Add State(s) to Queue__jki_lib_state_machine.vi"("State(s) in (\"\")"=w157, "State(s) at Back (\"\")"="Macro: start tests" ("State(s) at Back (\"\")")) -> ("States Out"=w156:string)  [unwired: 13 in]
      }
      frame "Data: Initialize" {
        w170 = T4 {"Test Sequence"=[{"TTrigger"=-130.0, "Direction"=enum."Falling", "TDelay"=0.0, "Type"=enum."No Test", "Pre-Log (s)"=0.0, "Duration (s)"=0.0, "Post-Log(s)"=0.0}, {"TTrigger"=-80.0, "Direction"=enum."Rising", "TDelay"=0.0, "Type"=enum."Heater Test", "Pre-Log (s)"=10.0, "Duration (s)"=15.0, "Post-Log(s)"=10.0}], "ActuationsPerLoop"=2, "Temperature Log Period(ms)"=1000, "PSU  Log Period (ms)"=100, "Diode Test Options"={"Temp.Tol"=0.0, "Max IDark"=[], "Min ILight"=[], "Min TEC \nCurrent"=0.0, "Max TEC \nCurrent"=0.0}, "Heater Test Options"={"Heater Nominal Voltage (A)"=0.67, "Heater Voltage Tolerance (%)"=20.0}}  # TestDefinitions
        w171 = path ""  # LogFilePath
        w172 = T5 {"TTrigger"=-130.0, "Direction"=enum."Falling", "TDelay"=0.0, "Type"=enum."No Test", "Pre-Log (s)"=10.0, "Duration (s)"=30.0, "Post-Log(s)"=100.0}  # CurrentTest
        w173 = 0  # CurrentCycle
        w174 = path ""  # TopFolderPath
        w175 = 0  # TestNumber
        w176 = T14 {"Current VI Reference"=refnum, "Close Panel on Exit?"=FALSE}  # Core
        w177 = ""  # TestPrefix
        # "Data names and types of shift register data are defined by this bundle."
        # "Initialize the shift-register data, here.\n(data names are defined by what you wire into the bundle function)"
        n70 = Bundle("Core"=w176, "CurrentCycle"=w173, "TestNumber"=w175, "TopFolderPath"=w174, "LogFilePath"=w171, "TestPrefix"=w177, "CurrentTest"=w172, "TestDefinitions"=w170) -> (w179:T12)  [unwired: 1 in]
        n71 = call <vilib>:"Add State(s) to Queue__jki_lib_state_machine.vi"("State(s) in (\"\")"=w181) -> ("States Out"=w180:string)  [unwired: 14 in]
      }
      frame "Data: Cleanup" {
        # "Cleanup any data and references, here.\n(this is called automatically, by the Macro: Exit)"
        n72 = Unbundle By Name(w182) -> ("Core.Current VI Reference"=w185:refnum<vi>)
        n73 = Close Reference(reference=w185, error in (no error)=w184) -> (error out=w183:errorcluster)
        n74 = call <vilib>:"Add State(s) to Queue__jki_lib_state_machine.vi"("State(s) in (\"\")"=w187) -> ("States Out"=w186:string)  [unwired: 14 in]
      }
      frame "---------- UI ----------" {
        # "Do not put any code in this frame.\n(It is a separator no-op. You can make a copy of this frame to create a new UI frame)"
        n75 = call <vilib>:"Add State(s) to Queue__jki_lib_state_machine.vi"("State(s) in (\"\")"=w191) -> ("States Out"=w190:string)  [unwired: 14 in]
      }
      frame "UI: Wait for Next1" {
        # "Wait for user to press OK button#1"
        n76 = while {
          stop <- "Next1" stop-if-true
          # "Wait for OK button"
        }
        n77 = call <vilib>:"Add State(s) to Queue__jki_lib_state_machine.vi"("State(s) in (\"\")"=w195) -> ("States Out"=w194:string)  [unwired: 14 in]
      }
      frame "UI: Initialize" {
        w200 = ""
        w201 = FALSE ("Heater Enable")
        # "Store ref to Message Log in global"
        # "Initialize the User Interface, here.\n(this is called automatically, by the Macro: Initialize)"
        n78 = control-ref of="Messages"() -> (w198:refnum<vi>)
        n79 = global write "Globals.vi" "LogMessagesRef"(w198) -> ()
        n80 = property on="TED" class="WFChart (strict)"("History Data"=waveform(dbl)[][] []) -> ()  [unwired: 2 in, 2 out]
        n81 = property on="Diode Currents" class="WFChart (strict)"("History Data"=waveform(dbl)[][] []) -> ()  [unwired: 2 in, 2 out]
        n82 = property on="Main Tabs" class="TabCtl (strict)"("Value"=T1."Setup" ("Main Tabs")) -> ()  [unwired: 2 in, 2 out]
        n83 = local write "LED_Illuminate"(w201) -> ()
        n84 = local write "LED_Stimulate"(w201) -> ()
        n85 = local write "PSU Enable"(w201) -> ()
        n86 = local write "Heater Enable"(w201) -> ()
        n87 = call <vilib>:"Add State(s) to Queue__jki_lib_state_machine.vi"("State(s) in (\"\")"=w207) -> ("States Out"=w206:string)  [unwired: 14 in]
        "Status" <- w200
        "Master Logging" <- w201
        "HTR On" <- w201
        "HTR Log" <- w201
        "ACT Logging" <- w201
        "HTR_Fault" <- w201
        "TVC_StopAfterCycle" <- w201
        "ACT Fault" <- w201
        "Messages" <- w200
        "TEC Faults" <- bool[] [FALSE, FALSE] ("TEC Faults")
      }
      frame "UI: Uninitialize" {
        w211 = FALSE ("PSU Enable")
        # "Cleanup the User Interface, here.\n(this is called automatically, by the Macro: Exit)"
        n88 = property on="Status" class="Str"(error in=w209, "Value"="Tests Finished" ("Status")) -> (error out=w208:errorcluster)  [unwired: 1 in, 1 out]
        n89 = local write "PSU Enable"(w211) -> ()
        n90 = local write "Master Logging"(w211) -> ()
        n91 = local write "Heater Enable"(w211) -> ()
        n92 = local write "HTR Log"(w211) -> ()
        n93 = local write "ACT Logging"(w211) -> ()
        n94 = call <vilib>:"Add State(s) to Queue__jki_lib_state_machine.vi"("State(s) in (\"\")"=w214) -> ("States Out"=w213:string)  [unwired: 14 in]
      }
      frame "UI: Status" {
        # "Put status information on screen"
        n95 = property on="Status" class="Str"(error in=w217, "Value"=w215) -> (error out=w216:errorcluster)  [unwired: 1 in, 1 out]
        n96 = call <vilib>:"Add State(s) to Queue__jki_lib_state_machine.vi"("State(s) in (\"\")"=w220) -> ("States Out"=w219:string)  [unwired: 14 in]
      }
      frame "UI: Set Datasockets" {
        # "Use control references to point datasocket URLs to local host or TVC machine"
        n97 = control-ref of="TED"() -> (w235:refnum<vi>)
        n98 = control-ref of="Diode Currents"() -> (w223:refnum<vi>)
        n99 = control-ref of="Heater Enable"() -> (w229:refnum<vi>)
        n100 = control-ref of="PSU Enable"() -> (w228:refnum<vi>)
        n101 = control-ref of="LED_Illuminate"() -> (w222:refnum<vi>)
        n102 = control-ref of="LED_Stimulate"() -> (w221:refnum<vi>)
        n103 = control-ref of="TVC_CyclesRemaining"() -> (w230:refnum<vi>)
        n104 = control-ref of="TVC_CycleNumber"() -> (w226:refnum<vi>)
        n105 = control-ref of="TVC_Temperatures"() -> (w231:refnum<vi>)
        n106 = control-ref of="TLUP_Temperatures"() -> (w227:refnum<vi>)
        n107 = control-ref of="Heater Monitor"() -> (w233:refnum<vi>)
        n108 = control-ref of="PSU_Monitor"() -> (w234:refnum<vi>)
        n109 = control-ref of="TEC On"() -> (w236:refnum<vi>)
        n110 = Build Array(w231, w227, w230, w226, w233, w229, w234, w228, w235, w236, w223, w222, w221) -> (w232:refnum<vi>[])
        n111 = for {
          tunnel: w232 -> [w251] mode=indexing
          tunnel: [w242] -> w224
          tunnel: w225 -> [w240]
          # "Use control references to point datasocket URLs to local host or TVC machine"
          n112 = property on="Server IP" class="Ring (strict)"() -> ("RingText.Text"=w250:string)  [unwired: 2 in, 2 out]
          n113 = property class="Ctl"(reference=w251, error in=w240) -> (reference out=w244:refnum<vi>, error out=w241:errorcluster, "DtSktURL"=w247:string)
          n114 = Concatenate Strings("dstp://" ("string"), w250, "/" ("string")) -> (w246:string)
          n115 = call <vilib>:"Search and Replace Pattern.vi"("string"=w247, "regular expression (\"\")"="dstp://.*/" ("regular expression (\"\")"), "replace string (\"\")"=w246) -> ("result string"=w243:string)  [unwired: 2 in, 1 out]
          n116 = property class="Ctl"(reference=w244, error in=w241, "DtSktURL"=w243) -> (error out=w242:errorcluster)  [unwired: 1 out]
        }
        n117 = call <vilib>:"Add State(s) to Queue__jki_lib_state_machine.vi"("State(s) in (\"\")"=w239) -> ("States Out"=w238:string)  [unwired: 14 in]
      }
      frame "UI: Cursor Set" {
        # "Argument"
        # "Set and Unset Cursor Busy.\n(Usage: \"UI: Cursor Set >> Busy|Idle\")"
        n118 = case shown="\"Idle\", Default" w252 {
          tunnel: w254 -> [w259 w261]
          tunnel: [w258 w260] -> w253
          frame "Idle", Default {
            n119 = call <vilib>:"Unset Busy.vi"("error in (no error)"=w259) -> ("error out"=w258:errorcluster)  [unwired: 10 in]
          }
          frame "Busy" {
            n120 = call <vilib>:"Set Busy.vi"("error in (no error)"=w261) -> ("error out"=w260:errorcluster)  [unwired: 9 in, 1 out]
          }
        }
        n121 = call <vilib>:"Add State(s) to Queue__jki_lib_state_machine.vi"("State(s) in (\"\")"=w257) -> ("States Out"=w256:string)  [unwired: 14 in]
      }
      frame "UI: Front Panel State" {
        # "Argument"
        # "Set Front Panel Open or Closed\n(Usage: \"UI: Front Panel State >> Open|Close\")"
        n122 = Unbundle By Name(w264) -> ("Core.Current VI Reference"=w263:refnum<vi>)
        n123 = case shown="\"Minimize\", \"Minimized\"" w262 {
          tunnel: w266 -> [w274 w289 w300 w313 w326]
          tunnel: [w276 w290 w302 w315 w328] -> w265
          tunnel: w263 -> [w275 w287 w301 w314 w327]
          frame "Open", "Standard", Default {
            w269 = T9."Standard" ("State")
            n124 = property class="VI"(reference=w275, error in=w274) -> (reference out=w272:refnum<vi>, error out=w273:errorcluster, "FP.State"=w271:T9)
            n125 = Not Equal?(x=w271, y=w269) -> (x != y?=w270:bool)
            n126 = case shown="True" w270 {
              tunnel: [w280 w282] -> w276
              tunnel: w273 -> [w279 w282]
              tunnel: w272 -> [w278 _]
              tunnel: w269 -> [w277 _]
              frame True {
                n127 = invoke class="VI" method="FP.Open"(reference=w278, error in=w279, "Activate"=TRUE, "State"=w277) -> (error out=w280:errorcluster)  [unwired: 1 in, 4 out]
              }
              frame False {
              }
            }
          }
          frame "Close", "Closed" {
            n128 = property class="VI"(reference=w287, error in=w289) -> (reference out=w286:refnum<vi>, error out=w288:errorcluster, "FP.State"=w284:T9)
            n129 = Not Equal?(x=w284, y=T9."Closed" ("Front Panel Window:State")) -> (x != y?=w283:bool)
            n130 = case shown="True" w283 {
              tunnel: [w291 w294] -> w290
              tunnel: w288 -> [w291 w293]
              tunnel: w286 -> [_ w292]
              frame False {
              }
              frame True {
                n131 = invoke class="VI" method="FP.Close"(reference=w292, error in=w293) -> (error out=w294:errorcluster)  [unwired: 1 in, 2 out]
              }
            }
          }
          frame "Hidden", "Hide" {
            w295 = T9."Hidden" ("State")
            n132 = property class="VI"(reference=w301, error in=w300) -> (reference out=w298:refnum<vi>, error out=w299:errorcluster, "FP.State"=w297:T9)
            n133 = Not Equal?(x=w297, y=w295) -> (x != y?=w296:bool)
            n134 = case shown="True" w296 {
              tunnel: [w306 w307] -> w302
              tunnel: w299 -> [w305 w307]
              tunnel: w298 -> [w304 _]
              tunnel: w295 -> [w303 _]
              frame True {
                n135 = invoke class="VI" method="FP.Open"(reference=w304, error in=w305, "State"=w303) -> (error out=w306:errorcluster)  [unwired: 2 in, 4 out]
              }
              frame False {
              }
            }
          }
          frame "Minimize", "Minimized" {
            w308 = T9."Minimized" ("State")
            n136 = property class="VI"(reference=w314, error in=w313) -> (reference out=w311:refnum<vi>, error out=w312:errorcluster, "FP.State"=w310:T9)
            n137 = Not Equal?(x=w310, y=w308) -> (x != y?=w309:bool)
            n138 = case shown="True" w309 {
              tunnel: [w319 w320] -> w315
              tunnel: w312 -> [w318 w320]
              tunnel: w311 -> [w317 _]
              tunnel: w308 -> [w316 _]
              frame True {
                n139 = invoke class="VI" method="FP.Open"(reference=w317, error in=w318, "State"=w316) -> (error out=w319:errorcluster)  [unwired: 2 in, 4 out]
              }
              frame False {
              }
            }
          }
          frame "Maximize", "Maximized" {
            w321 = T9."Maximized" ("State")
            n140 = property class="VI"(reference=w327, error in=w326) -> (reference out=w324:refnum<vi>, error out=w325:errorcluster, "FP.State"=w323:T9)
            n141 = Not Equal?(x=w323, y=w321) -> (x != y?=w322:bool)
            n142 = case shown="True" w322 {
              tunnel: [w332 w333] -> w328
              tunnel: w325 -> [w331 w333]
              tunnel: w324 -> [w330 _]
              tunnel: w321 -> [w329 _]
              frame True {
                n143 = invoke class="VI" method="FP.Open"(reference=w330, error in=w331, "State"=w329) -> (error out=w332:errorcluster)  [unwired: 2 in, 4 out]
              }
              frame False {
              }
            }
          }
        }
        n144 = call <vilib>:"Add State(s) to Queue__jki_lib_state_machine.vi"("State(s) in (\"\")"=w268) -> ("States Out"=w267:string)  [unwired: 14 in]
      }
      frame "---------- Macro ----------" {
        # "Do not put any code in this frame.\n(It is a separator no-op. You can make a copy of this frame to create a new Macro frame)"
        n145 = call <vilib>:"Add State(s) to Queue__jki_lib_state_machine.vi"("State(s) in (\"\")"=w337) -> ("States Out"=w336:string)  [unwired: 14 in]
      }
      frame "Macro: Initialize" {
        # "Initialization Macro\n(This is called once, when the VI starts)"
        n146 = call <vilib>:"Add State(s) to Queue__jki_lib_state_machine.vi"("State(s) in Front (\"\")"="Data: Initialize\nInitialize Core Data\nUI: Initialize\nUI: Front Panel State >> Open\nUI: Set Datasockets\nData: Load Definitions\nHardware: Setup TVC\nUI: Status >>Setup - Fill in fields and press Next to Continue\nUI: Wait for Next1\nData: Check Folders\nHardware: Check Camera\nUI: Status>> Review Hardware and Press Next to Continue\nHardware: Review\nUI: Status>> Review Test and Press Next to Start Test Sequence\nData: Review Tests ", "State(s) in (\"\")"=w342) -> ("States Out"=w341:string)  [unwired: 13 in]
      }
      frame "Macro: Stabilise" {
        # "stabilise"
        # "Stabilise:\nCall routine to allow system to stabilise"
        n147 = Decimal String To Number(string=w347) -> (number=w346:i32)  [unwired: 2 in, 1 out]
        n148 = property on="Status" class="Str"(error in=w344, "Value"="Stabilisation delay" ("Status")) -> (error out=w345:errorcluster)  [unwired: 1 in, 1 out]
        n149 = control-ref of="DelayRemaining"() -> (w349:refnum<vi>)
        n150 = Multiply(x=60.0 ("y"), y=w346) -> (x*y=w351:dbl)
        n151 = call "DelayTimer.vi"("Formatted \nTime Ref"=w349, "FormatString"="Stabilise: %M:%S", "error in (no error)"=w345, "Delay(s)"=w351) -> ("error out"=w348:errorcluster)  [unwired: 7 in]
        n152 = call <vilib>:"Add State(s) to Queue__jki_lib_state_machine.vi"("State(s) in (\"\")"=w355) -> ("States Out"=w354:string)  [unwired: 14 in]
      }
      frame "Macro: start tests" {
        n153 = property on="Master Logging" class="Bool (strict)"(error in=w365, "Value"=TRUE ("Graphing")) -> (error out=w369:errorcluster)  [unwired: 1 in, 1 out]
        n154 = property on="Temperatures" class="WFChart (strict)"(error in=w369, "History Data"=waveform(dbl)[] []) -> (error out=w368:errorcluster)  [unwired: 1 in, 1 out]
        n155 = Bundle By Name(cluster=w370, "CurrentCycle"=0, "TestNumber"=0 ("CurrentTest")) -> (w364:T12)
        n156 = property on="Main Tabs" class="TabCtl (strict)"(error in=w368, "Value"=T1."Operating" ("Main Tabs")) -> (error out=w359:errorcluster)  [unwired: 1 in, 1 out]
        n157 = call "WriteLogFile.vi"("error in (no error)"=w359, "Message"="Test Sequence Starts") -> ("error out"=w358:errorcluster)  [unwired: 9 in]
        n158 = call <vilib>:"Add State(s) to Queue__jki_lib_state_machine.vi"("State(s) in (\"\")"=w372, "State(s) at Back (\"\")"="Macro: Wait For Trigger" ("State(s) at Back (\"\")")) -> ("States Out"=w371:string)  [unwired: 13 in]
        "TVC_CyclesRemaining" <- "Cycles To Run"
      }
      frame "Macro: Wait For Trigger" {
        n159 = Unbundle By Name(w374) -> ("TestNumber"=w376:i32)
        n160 = local read "TestDefinition"() -> (w380:T4)
        n161 = Unbundle By Name(w380) -> ("Test Sequence"=w378:T5[])
        n162 = Array Size(array=w378) -> (size(s)=w377:i32)
        n163 = Greater Or Equal?(x=w376, y=w377) -> (x >= y?=w375:bool)
        n164 = case shown="False" w375 {
          tunnel: w382 -> [w401 w423]
          tunnel: [w387 w423] -> w381
          tunnel: [w397 "Macro: End Cycle"] -> w379
          tunnel: w378 -> [w396 _]
          tunnel: w376 -> [w395 _]
          tunnel: w374 -> [w394 w421]
          tunnel: [w393 w421] -> w373
          frame False {
            # "Not at end test yet, so wait for trigger"
            n165 = Index Array(array=w396, index=w395) -> (element=w392:T5)
            n166 = while {
              tunnel: w392 -> [w404]
              tunnel: [w411] -> w399
              tunnel: w401 -> [w409]
              tunnel: [w408] -> w386
              tunnel: [w402] -> w389
              stop <- w414 stop-if-true
              # "Pick temperature reading"
              # "Loop waiting for test condition"
              n167 = local read "TVC_Temperatures"() -> (w405:waveform(dbl)[])
              n168 = Unbundle By Name(w404) -> ("TTrigger"=w402:dbl, "Direction"=w410:enum16{"Rising", "Falling"}, "TDelay"=w411:dbl)
              n169 = Index Array(array=w405, index="ControlChannel") -> (element=w413:waveform(dbl))
              n170 = Unbundle By Name(w413) -> ("Y"=w412:dbl[])
              n171 = Index Array(array=w412) -> (element=w406:dbl)  [unwired: 1 in]
              n172 = call "Make Status Message.vi"("Direction"=w410, "TTrigger"=w402) -> ("Status Message"=w407:string)  [unwired: 9 in]
              n173 = case shown="\"Rising\", Default" w410 {
                tunnel: w406 -> [w416 w419]
                tunnel: w402 -> [w417 w420]
                tunnel: [w415 w418] -> w414
                frame "Rising", Default {
                  # "Trigger when TControl\n>=TTrigger"
                  n174 = Greater Or Equal?(x=w416, y=w417) -> (x >= y?=w415:bool)
                }
                frame "Falling" {
                  # "Trigger when TControl<TTrigger"
                  n175 = Less Or Equal?(x=w419, y=w420) -> (x <= y?=w418:bool)
                }
              }
              n176 = property on="Status" class="Str"(error in=w409, "Value"=w407) -> (error out=w408:errorcluster)  [unwired: 1 in, 1 out]
            }
            n177 = Bundle By Name(cluster=w394, "CurrentTest"=w392) -> (w393:T12)
            n178 = Format Into String(format string="Macro: stabilise>>%d", w399) -> (resulting string=w398:string)  [unwired: 2 in, 1 out]
            n179 = Concatenate Strings(w398, "\r\n", "Macro: Run Test") -> (w397:string)
            n180 = Format Into String(format string="Trigger at %.1fC reached", w389) -> (resulting string=w385:string)  [unwired: 2 in, 1 out]
            n181 = call "WriteLogFile.vi"("error in (no error)"=w386, "Message"=w385) -> ("error out"=w387:errorcluster)  [unwired: 9 in]
          }
          frame True {
            # "Tests finished"
          }
        }
        n182 = call <vilib>:"Add State(s) to Queue__jki_lib_state_machine.vi"("State(s) in (\"\")"=w384, "State(s) at Back (\"\")"=w379) -> ("States Out"=w383:string)  [unwired: 13 in]
      }
      frame "Macro: Run Test" {
        n183 = Unbundle By Name(w438) -> ("CurrentTest.Type"=w431:T6, "CurrentTest.TTrigger"=w435:dbl)
        n184 = Not Equal?(x=TestType."No Test", y=w431) -> (x != y?=w436:bool)
        n185 = case shown="True" w436 {
          tunnel: [_ w469] -> w433
          tunnel: [_ w468] -> w432
          tunnel: w435 -> [_ w463]
          frame False {
            # "Don't create directory for null test"
          }
          frame True {
            # "Create Prefix for this test\nand make directory to store \nit in"
            n186 = local read "TopFolderPrefix"() -> (w470:string)
            n187 = local read "TopFolderPath"() -> (w467:path)
            n188 = Add(x="TVC_CycleNumber", y="StartCycle") -> (x+y=w464:i32)
            n189 = call "MakePrefix.vi"("TempPoint"=w463, "TempCycleNo"=w464, "FolderPrefix"=w470, "TopFolderPath"=w467) -> ("Prefix"=w468:string, "TestFolderPath"=w469:path)  [unwired: 6 in]
          }
        }
        n190 = Bundle By Name(cluster=w438, "TopFolderPath"=w433, "TestPrefix"=w432) -> (w434:T12)
        n191 = case shown="\"Diode Test\"" w431 {
          tunnel: "Macro: Run_" -> [w443 w450 w455 w461]
          tunnel: [w444 w448 w456 w462] -> w429
          tunnel: ["" w446 w452 w458] -> w425
          tunnel: "Preparing" -> [_ w445 w451 w457]
          frame "No Test", Default {
            n192 = Concatenate Strings(w443, "NULL" ("string")) -> (w444:string)
          }
          frame "Heater Test" {
            n193 = Concatenate Strings(w445, " Heater " ("string")) -> (w446:string)
            n194 = Concatenate Strings(w450, "HTR" ("string")) -> (w448:string)
          }
          frame "Actuation Test" {
            n195 = Concatenate Strings(w451, " Actuation " ("string")) -> (w452:string)
            n196 = Concatenate Strings(w455, "ACT" ("string")) -> (w456:string)
          }
          frame "Diode Test" {
            n197 = Concatenate Strings(w457, " Diode " ("string")) -> (w458:string)
            n198 = Concatenate Strings(w461, "DIODE" ("string")) -> (w462:string)
          }
        }
        n199 = Concatenate Strings(w425, "Test" ("string")) -> (w427:string)
        n200 = property on="Status" class="Str"("Value"=w427) -> ()  [unwired: 2 in, 2 out]
        n201 = call <vilib>:"Add State(s) to Queue__jki_lib_state_machine.vi"("State(s) in (\"\")"=w440, "State(s) at Back (\"\")"=w429) -> ("States Out"=w439:string)  [unwired: 13 in]
      }
      frame "Macro: Run_NULL" {
        # "NULL Test - Does nothing except increment test numbe and go back\nto wait for trigger"
        n202 = in-place {
          n203 = in-place-cluster #1(w476) -> ("TestNumber"=w480:i32)
          n204 = Increment(x=w480) -> (x+1=w479:i32)
          n205 = in-place-cluster #1("TestNumber"=w479) -> (w475:T12)
        }
        n206 = call "WriteLogFile.vi"("error in (no error)"=w472, "Message"="NULL test") -> ("error out"=w473:errorcluster)  [unwired: 9 in]
        n207 = call <vilib>:"Add State(s) to Queue__jki_lib_state_machine.vi"("State(s) in (\"\")"=w478, "State(s) at Back (\"\")"="Macro: Wait For Trigger" ("State(s) at Back (\"\")")) -> ("States Out"=w477:string)  [unwired: 13 in]
      }
      frame "Macro: Run_HTR" {
        # "Heater Test"
        n208 = local read "HTR_Fault"() -> (w481:bool)
        n209 = case shown="False" w481 {
          tunnel: w484 -> [w506 _]
          tunnel: [w497 w530] -> w483
          tunnel: w482 -> [w492 w531]
          frame False {
            # "These both refer to booleans relating\nto the heater.\nHTR Enable does the switching\nHTR On is a front panel mimic"
            # "Form heater log names"
            n210 = Unbundle By Name(w506) -> ("TopFolderPath"=w505:path, "TestPrefix"=w504:string, "CurrentTest"=w501:T5)
            n211 = local read "TestDefinition"() -> (w490:T4)
            n212 = property on="HTR Log" class="Bool (strict)"(error in=w492, "Value"=TRUE ("Heater Logging")) -> (error out=w493:errorcluster)  [unwired: 1 in, 1 out]
            n213 = Unbundle By Name(w490) -> ("PSU  Log Period (ms)"=w513:i64, "Temperature Log Period(ms)"=w514:i64)
            n214 = Concatenate Strings(w504, "Temp.xlsx" ("string")) -> (w510:string)
            n215 = Concatenate Strings(w504, "PSU.xlsx" ("string")) -> (w511:string)
            n216 = Build Path(base path=w505, name or relative path=w510) -> (appended path=w509:path)
            n217 = Build Path(base path=w505, name or relative path=w511) -> (appended path=w512:path)
            n218 = Unbundle By Name(w490) -> ("Heater Test Options"=w489:T8)
            n219 = control-ref of="HTR_Fault"() -> (w494:refnum<vi>)
            n220 = control-ref of="Status"() -> (w502:refnum<vi>)
            n221 = control-ref of="DelayRemaining"() -> (w503:refnum<vi>)
            n222 = control-ref of="Heater Monitor"() -> (w491:refnum<vi>)
            n223 = while {
              tunnel: w512 -> [w526]
              tunnel: w513 -> [w522]
              tunnel: w493 -> [_]
              stop <- w523 stop-if-true
              n224 = Wait Until Next ms Multiple(millisecond multiple=w522) -> ()  [unwired: 1 out]
              n225 = local read "Heater Monitor"() -> (w525:waveform(dbl)[])
              n226 = local read "PSU_Monitor"() -> (w524:waveform(dbl)[])
              n227 = local read "HTR Log"() -> (w528:bool)
              n228 = Not(x=w528) -> (.not. x?=w523:bool)
              n229 = Merge Signals(w525, w524) -> (w527:dynamicdata)
              n230 = call "Write Voltage and Current Log File"("Signals"=w527, "Flush? (T)"=w523, "Filename"=w526) -> ()  [unwired: 14 in, 3 out]
            }
            n231 = while {
              tunnel: w509 -> [w521]
              tunnel: w514 -> [w515]
              tunnel: w493 -> [_]
              stop <- w519 stop-if-true
              n232 = local read "TLUP_Temperatures"() -> (w517:waveform(dbl)[])
              n233 = local read "TVC_Temperatures"() -> (w518:waveform(dbl)[])
              n234 = Wait Until Next ms Multiple(millisecond multiple=w515) -> ()  [unwired: 1 out]
              n235 = local read "HTR Log"() -> (w516:bool)
              n236 = Not(x=w516) -> (.not. x?=w519:bool)
              n237 = Merge Signals(w518, w517) -> (w520:dynamicdata)
              n238 = call "Write Temperature Log File"("Signals"=w520, "Flush? (T)"=w519, "Filename"=w521) -> ()  [unwired: 14 in, 3 out]
            }
            n239 = control-ref of="Heater Enable"() -> (w500:refnum<vi>)
            n240 = control-ref of="HTR On"() -> (w495:refnum<vi>)
            n241 = call "HTR_Test.vi"("CurrentTest"=w501, "Status Ref"=w502, "HTR_Monitor Ref"=w491, "HTR_OnOff Ref"=w495, "Heater Test Options"=w489, "HTR Fault Ref"=w494, "error in (no error)"=w493, "DelayRemaining"=w503, "HTR_Enable Ref"=w500) -> ("error out"=w496:errorcluster)  [unwired: 6 in]
            n242 = property on="HTR Log" class="Bool (strict)"(error in=w496, "Value"=FALSE ("Heater Logging")) -> (error out=w497:errorcluster)  [unwired: 1 in, 1 out]
          }
          frame True {
            n243 = call "WriteLogFile.vi"("error in (no error)"=w531, "Message"="Heater Test Skipped due to previous fault") -> ("error out"=w530:errorcluster)  [unwired: 9 in]
          }
        }
        n244 = in-place {
          n245 = in-place-cluster #2(w484) -> ("TestNumber"=w533:i32)
          n246 = Increment(x=w533) -> (x+1=w532:i32)
          n247 = in-place-cluster #2("TestNumber"=w532) -> (w486:T12)
        }
        n248 = call <vilib>:"Add State(s) to Queue__jki_lib_state_machine.vi"("State(s) in (\"\")"=w488, "State(s) at Back (\"\")"="Macro: Wait For Trigger" ("State(s) at Back (\"\")")) -> ("States Out"=w487:string)  [unwired: 13 in]
      }
      frame "Macro: Run_DIODE" {
        w536 = "Diode Test Finish" ("Status")
        w537 = "Diode Test Start" ("Status")
        # "Form Diode log names"
        # "Start Logging before \nenabling Peltier"
        # "Run Diode Test"
        n249 = Unbundle By Name(w549) -> ("CurrentTest"=w543:T5)
        n250 = Unbundle By Name(w549) -> ("TopFolderPath"=w553:path, "TestPrefix"=w554:string)
        n251 = property on="Status" class="Str"(error in=w561, "Value"=w537) -> (error out=w550:errorcluster)  [unwired: 1 in, 1 out]
        n252 = local read "TestDefinition"() -> (w534:T4)
        n253 = call "WriteLogFile.vi"("error in (no error)"=w550, "Message"=w537) -> ("error out"=w551:errorcluster)  [unwired: 9 in]
        n254 = in-place {
          n255 = in-place-cluster #3(w549) -> ("TestNumber"=w576:i32)
          n256 = Increment(x=w576) -> (x+1=w575:i32)
          n257 = in-place-cluster #3("TestNumber"=w575) -> (w563:T12)
        }
        n258 = Unbundle By Name(w534) -> ("Temperature Log Period(ms)"=w560:i64)
        n259 = property on="Diode Logging" class="Bool (strict)"(error in=w551, "Value"=TRUE ("Heater PSU")) -> (error out=w541:errorcluster)  [unwired: 1 in, 1 out]
        n260 = Unbundle By Name(w534) -> ("Diode Test Options"=w535:T7)
        n261 = Concatenate Strings(w554, "Diode.xlsx" ("string")) -> (w559:string)
        n262 = Build Path(base path=w553, name or relative path=w559) -> (appended path=w558:path)
        n263 = control-ref of="Diode Currents"() -> (w547:refnum<vi>)
        n264 = control-ref of="LED_Stimulate"() -> (w545:refnum<vi>)
        n265 = control-ref of="DelayRemaining"() -> (w546:refnum<vi>)
        n266 = control-ref of="TED Status"() -> (w542:refnum<vi>)
        n267 = control-ref of="TEC Faults"() -> (w548:refnum<vi>)
        n268 = while {
          tunnel: w558 -> [w574]
          tunnel: w541 -> [_]
          tunnel: w560 -> [w568]
          stop <- w572 stop-if-true
          # "Diode Logging"
          n269 = Wait Until Next ms Multiple(millisecond multiple=w568) -> ()  [unwired: 1 out]
          n270 = local read "Diode Logging"() -> (w569:bool)
          n271 = local read "TLUP_Temperatures"() -> (w570:waveform(dbl)[])
          n272 = local read "TVC_Temperatures"() -> (w571:waveform(dbl)[])
          n273 = local read "Diode Currents"() -> (w567:waveform(dbl)[])
          n274 = local read "TED"() -> (w566:waveform(dbl)[])
          n275 = Not(x=w569) -> (.not. x?=w572:bool)
          n276 = Merge Signals(w566, w567, w571, w570) -> (w573:dynamicdata)
          n277 = call "Write Diode Log File"("Signals"=w573, "Flush? (T)"=w572, "Filename"=w574) -> ()  [unwired: 14 in, 3 out]
        }
        n278 = control-ref of="TEC On"() -> (w544:refnum<vi>)
        n279 = call "DiodeTestAndCheck.vi"("Diode Test Options"=w535, "Stimulus_LED"=w545, "DelayStr Ref"=w546, "Diode Currents"=w547, "TEC Faults Ref"=w548, "CurrentTest"=w543, "Peltier_OnOffs"=w544, "error in (no error)"=w541, "TED Status"=w542) -> ("error out"=w540:errorcluster)  [unwired: 6 in]
        n280 = property on="Diode Logging" class="Bool (strict)"(error in=w540, "Value"=FALSE ("Heater Logging")) -> (error out=w552:errorcluster)  [unwired: 1 in, 1 out]
        n281 = property on="Status" class="Str"(error in=w552, "Value"=w536) -> (error out=w538:errorcluster)  [unwired: 1 in, 1 out]
        n282 = call "WriteLogFile.vi"("error in (no error)"=w538, "Message"=w536) -> ("error out"=w539:errorcluster)  [unwired: 9 in]
        n283 = call <vilib>:"Add State(s) to Queue__jki_lib_state_machine.vi"("State(s) in (\"\")"=w565, "State(s) at Back (\"\")"="Macro: Wait For Trigger" ("State(s) at Back (\"\")")) -> ("States Out"=w564:string)  [unwired: 13 in]
      }
      frame "Macro: Run_ACT" {
        # "ACT Test - Runs actuation test"
        n284 = local read "ACT Fault"() -> (w577:bool)
        n285 = case shown="False" w577 {
          tunnel: w580 -> [w599 _]
          tunnel: w579 -> [w595 w660]
          tunnel: [w588 w661] -> w578
          frame False {
            w589 = TRUE ("LED_Illuminate")
            w585 = "Actuation Test Start" ("Status")
            # "Test storage Directory"
            # "TestPrefix"
            n286 = local read "TestDefinition"() -> (w596:T4)
            n287 = property on="Status" class="Str"(error in=w595, "Value"=w585) -> (error out=w592:errorcluster)  [unwired: 1 in, 1 out]
            n288 = Unbundle By Name(w599) -> ("TopFolderPath"=w597:path, "TestPrefix"=w598:string, "CurrentTest"=w594:T5)
            n289 = call "WriteLogFile.vi"("error in (no error)"=w592, "Message"=w585) -> ("error out"=w593:errorcluster)  [unwired: 9 in]
            n290 = Unbundle By Name(w596) -> ("ActuationsPerLoop"=w600:i32)
            n291 = property on="LED_Illuminate" class="Bool (strict)"(error in=w593, "Value"=w589) -> (error out=w590:errorcluster)  [unwired: 1 in, 1 out]
            n292 = property on="PSU Enable" class="Bool (strict)"(error in=w590, "Value"=w589) -> (error out=w591:errorcluster)  [unwired: 1 in, 1 out]
            n293 = for {
              N: w600 -> [_]
              shift-right: [w604] -> w587
              shift-left: w591 -> [w608]
              tunnel: w596 -> [w610]
              tunnel: w598 -> [w609]
              tunnel: w597 -> [w606]
              tunnel: w594 -> [w607]
              i -> [w605]
              stop <- w604 stop-if-true
              n294 = local read "ACT Fault"() -> (w603:bool)
              n295 = case shown="False" w603 {
                tunnel: w610 -> [w631 _]
                tunnel: w609 -> [w630 _]
                tunnel: w608 -> [w628 w658]
                tunnel: w607 -> [w620 _]
                tunnel: w606 -> [w619 _]
                tunnel: w605 -> [w618 w654]
                tunnel: [w614 w657] -> w604
                frame False {
                  # "Add Actuation\nto TestPrefix"
                  n296 = Format Into String(format string="A%d_", initial string=w630, w618) -> (resulting string=w621:string)  [unwired: 1 in, 1 out]
                  n297 = local read "Path to Actuation Script"() -> (w624:path)
                  n298 = property on="ACT Logging" class="Bool (strict)"(error in=w628, "Value"=TRUE ("Actuation Logging")) -> (error out=w627:errorcluster)  [unwired: 1 in, 1 out]
                  n299 = Unbundle By Name(w631) -> ("PSU  Log Period (ms)"=w633:i64, "Temperature Log Period(ms)"=w632:i64)
                  n300 = local read "Camera"() -> (w623:string)
                  n301 = Concatenate Strings(w621, "PSU.xlsx" ("string")) -> (w637:string)
                  n302 = control-ref of="DelayRemaining"() -> (w626:refnum<vi>)
                  n303 = Concatenate Strings(w621, "Temp.xlsx" ("string")) -> (w639:string)
                  n304 = Build Path(base path=w619, name or relative path=w637) -> (appended path=w636:path)
                  n305 = Build Path(base path=w619, name or relative path=w639) -> (appended path=w638:path)
                  n306 = while {
                    tunnel: w638 -> [w648]
                    tunnel: w627 -> [_]
                    tunnel: w632 -> [w642]
                    stop <- w646 stop-if-true
                    # "write log file, \nbuffer to memory\nflush on exit"
                    # "write Temperature log"
                    n307 = Wait Until Next ms Multiple(millisecond multiple=w642) -> ()  [unwired: 1 out]
                    n308 = local read "TLUP_Temperatures"() -> (w643:waveform(dbl)[])
                    n309 = local read "TVC_Temperatures"() -> (w644:waveform(dbl)[])
                    n310 = local read "ACT Logging"() -> (w645:bool)
                    n311 = Not(x=w645) -> (.not. x?=w646:bool)
                    n312 = Merge Signals(w644, w643) -> (w647:dynamicdata)
                    n313 = call "Write Actuation Temperature Log"("Signals"=w647, "Flush? (T)"=w646, "Filename"=w648) -> ()  [unwired: 14 in, 3 out]
                  }
                  n314 = local read "FFMPEG exe"() -> (w625:path)
                  n315 = call "ACT_Test.vi"("CurrentTest"=w620, "Path to Actuation Script"=w624, "VideoSave Directory"=w619, "Path to FFMPEG"=w625, "DelayStr Ref"=w626, "Test Prefix"=w621, "error in (no error)"=w627, "Video Camera"=w623, "Actuation"=w618, "COM Port"="COM Port") -> ("return code"=w612:i32, "error out"=w615:errorcluster)  [unwired: 4 in]
                  n316 = Equal?(x=w612, y=1) -> (x = y?=w617:bool)
                  n317 = Equal To 0?(x=w612) -> (x = 0?=w611:bool)
                  n318 = while {
                    tunnel: w636 -> [w652]
                    tunnel: w627 -> [_]
                    tunnel: w633 -> [w649]
                    stop <- w650 stop-if-true
                    # "write log file, \nbuffer to memory\nflush on exit"
                    # "write Board PSU log"
                    n319 = Wait Until Next ms Multiple(millisecond multiple=w649) -> ()  [unwired: 1 out]
                    n320 = local read "ACT Logging"() -> (w651:bool)
                    n321 = local read "PSU_Monitor"() -> (w653:waveform(dbl)[])
                    n322 = Not(x=w651) -> (.not. x?=w650:bool)
                    n323 = call "Write Actuation PSU Log"("Signals"=w653, "Flush? (T)"=w650, "Filename"=w652) -> ()  [unwired: 14 in, 3 out]
                  }
                  n324 = flat-sequence {
                    tunnel: w615 -> [_]
                    tunnel: w615 -> [_]
                    frame #0 {
                      n325 = property on="ACT Logging" class="Bool (strict)"("Value"=FALSE ("Actuation Logging")) -> ()  [unwired: 2 in, 2 out]
                    }
                  }
                  n326 = local write "ACT Fault"(w617) -> ()
                  n327 = call "WriteLogFile.vi"("Write?"=w611, "error in (no error)"=w615, "Message"="Actuation Completed") -> ("error out"=w614:errorcluster)  [unwired: 8 in]
                }
                frame True {
                  n328 = Format Into String(format string="Actuation #%d cancelled due to previous error", w654) -> (resulting string=w656:string)  [unwired: 2 in, 1 out]
                  n329 = call "WriteLogFile.vi"("error in (no error)"=w658, "Message"=w656) -> ("error out"=w657:errorcluster)  [unwired: 9 in]
                }
              }
            }
            n330 = flat-sequence {
              tunnel: w587 -> [_]
              frame #0 {
                n331 = property on="LED_Illuminate" class="Bool (strict)"("Value"=FALSE ("LED_Illuminate")) -> ()  [unwired: 2 in, 2 out]
                n332 = property on="PSU Enable" class="Bool (strict)"("Value"=FALSE ("PSU Enable")) -> ()  [unwired: 2 in, 2 out]
              }
            }
            n333 = call "WriteLogFile.vi"("error in (no error)"=w587, "Message"="Actuation Test Finished") -> ("error out"=w588:errorcluster)  [unwired: 9 in]
          }
          frame True {
            n334 = call "WriteLogFile.vi"("error in (no error)"=w660, "Message"="Actuation Test Skipped due to previous error") -> ("error out"=w661:errorcluster)  [unwired: 9 in]
          }
        }
        n335 = in-place {
          n336 = in-place-cluster #4(w580) -> ("TestNumber"=w663:i32)
          n337 = Increment(x=w663) -> (x+1=w662:i32)
          n338 = in-place-cluster #4("TestNumber"=w662) -> (w582:T12)
        }
        n339 = call <vilib>:"Add State(s) to Queue__jki_lib_state_machine.vi"("State(s) in (\"\")"=w584, "State(s) at Back (\"\")"="Macro: Wait For Trigger" ("State(s) at Back (\"\")")) -> ("States Out"=w583:string)  [unwired: 13 in]
      }
      frame "Macro: End Cycle" {
        n340 = Unbundle By Name(w667) -> ("CurrentCycle"=w666:i32)
        n341 = in-place {
          in-place-border: [w674] -> w670
          n342 = in-place-cluster #5(w667) -> ("CurrentCycle"=w679:i32)  [unwired: 1 out]
          n343 = Increment(x=w679) -> (x+1=w675:i32)
          n344 = local read "Cycles To Run"() -> (w678:i32)
          n345 = Greater Or Equal?(x=w675, y=w678) -> (x >= y?=w677:bool)
          n346 = case shown="False" w677 {
            tunnel: [0 _] -> w676
            tunnel: ["Macro: Wait For Trigger" "Macro: Exit"] -> w674
            frame False {
            }
            frame True {
            }
          }
          n347 = in-place-cluster #5("CurrentCycle"=w675, "TestNumber"=w676) -> (w671:T12)
        }
        n348 = Format Into String(format string="Test Cycle %d finished" ("Log Message"), w666) -> (resulting string=w664:string)  [unwired: 2 in, 1 out]
        n349 = call "WriteLogFile.vi"("error in (no error)"=w669, "Message"=w664) -> ("error out"=w668:errorcluster)  [unwired: 9 in]
        n350 = call <vilib>:"Add State(s) to Queue__jki_lib_state_machine.vi"("State(s) in (\"\")"=w673, "State(s) at Back (\"\")"=w670) -> ("States Out"=w672:string)  [unwired: 13 in]
      }
      frame "Macro: AbortEndOfCycle" {
        n351 = call "WriteLogFile.vi"("error in (no error)"=w687, "Message"="Aborting at end of TVC Cycle" ("Log Message")) -> ("error out"=w686:errorcluster)  [unwired: 9 in]
        n352 = local write "TVC_StopAfterCycle"(TRUE ("TVC_StopAfterCycle")) -> ()
        n353 = call <vilib>:"Add State(s) to Queue__jki_lib_state_machine.vi"("State(s) in (\"\")"=w689) -> ("States Out"=w688:string)  [unwired: 14 in]
      }
      frame "Macro: Exit" {
        # "Exit Macro\n(This is called once, when the VI exits)"
        n354 = Unbundle By Name(w696) -> ("Core.Close Panel on Exit?"=w691:bool)
        n355 = call <vilib>:"Conditional State String__jki_lib_state_machine.vi"("Do State(s)?"=w691, "State"="UI: Front Panel State >> Close") -> ("State Out"=w690:string)  [unwired: 7 in]
        n356 = call <vilib>:"Add State(s) to Queue__jki_lib_state_machine.vi"("State(s) in (\"\")"=w690, "State(s) at Back (\"\")"="UI: Uninitialize\nData: Cleanup\nExit") -> ("States Out"=w694:string)  [unwired: 13 in]
        n357 = call <vilib>:"Add State(s) to Queue__jki_lib_state_machine.vi"("State(s) in Front (\"\")"=w694, "State(s) in (\"\")"=w698) -> ("States Out"=w697:string)  [unwired: 13 in]
      }
      frame "---------- Hardware ----------" {
        # "Template Separator\n(You can make a copy of, or modify, this frame)"
        n358 = call <vilib>:"Add State(s) to Queue__jki_lib_state_machine.vi"("State(s) in (\"\")"=w702) -> ("States Out"=w701:string)  [unwired: 14 in]
      }
      frame "Hardware: Setup TVC" {
        n359 = while {
          tunnel: ["TVC_Temperatures"] -> w706
          tunnel: [w718] -> w708
          tunnel: w704 -> [w717]
          stop <- w720 stop-if-true
          # "Wait Until TVC Temperatures connected"
          n360 = property on="TVC_Temperatures" class="Arr (strict)"(error in=w717) -> (error out=w718:errorcluster, "DtSktStatus"=w723:T15)  [unwired: 1 in, 1 out]
          n361 = Unbundle By Name(w723) -> ("Code"=w722:T11)
          n362 = Equal?(x=w722, y=T11."Active") -> (x = y?=w720:bool)
        }
        n363 = for {
          tunnel: w706 -> [w716] mode=indexing
          tunnel: "NI_ChannelName" ("name") -> [w715]
          tunnel: [w714] -> w707 mode=indexing
          tunnel: w708 -> [w713]
          tunnel: [w712] -> w703
          n364 = Get Waveform Attribute(4:w713, 5:w715, 6:w715, 7:w716) -> (0:w712:errorcluster, 1:w714:string)  [unwired: 2 out]
        }
        "ChannelNames" <- w707
        n365 = property on="ControlChannel" class="Ring (strict)"("Strings []"=w707) -> ()  [unwired: 2 in, 2 out]
        n366 = call <vilib>:"Add State(s) to Queue__jki_lib_state_machine.vi"("State(s) in (\"\")"=w711) -> ("States Out"=w710:string)  [unwired: 14 in]
      }
      frame "Hardware: Check Camera" {
        # "check FFMPeg exists"
        n367 = call <vilib>:"Check if File or Folder Exists.vi"("error in (no error)"=w728, "path"="FFMPEG exe") -> ("error out"=w731:errorcluster, "file or folder exists?"=w732:bool)  [unwired: 7 in, 1 out]
        n368 = Select(t=w731, s=w732, f=errorcluster {"status"=TRUE, "code"=5001, "source"="Video Device Not Found"} ("error constant")) -> (s? t:f=w730:errorcluster)
        n369 = call "FindVideoDevices.vi"("error in (no error)"=w730, "Path to FFMPEG"="FFMPEG exe") -> ("error out"=w726:errorcluster, "Video Devices"=w733:string[])  [unwired: 8 in]
        n370 = property on="Video Camera" class="Ring (strict)"("Strings []"=w733) -> ()  [unwired: 2 in, 2 out]
        n371 = property on="Status" class="Str"(error in=w726, "Value"="Camera OK" ("State(s) at Back (\"\")")) -> (error out=w725:errorcluster)  [unwired: 1 in, 1 out]
        n372 = call <vilib>:"Add State(s) to Queue__jki_lib_state_machine.vi"("State(s) in (\"\")"=w736) -> ("States Out"=w735:string)  [unwired: 14 in]
      }
      frame "Hardware: Review" {
        # "save text from Video Camera \ncontrol to pass into capture routine"
        n373 = property on="Main Tabs" class="TabCtl (strict)"(error in=w742, "Value"=T1."Hardware" ("Main Tabs")) -> (error out=w741:errorcluster)  [unwired: 1 in, 1 out]
        n374 = while {
          tunnel: w741 -> [w747]
          tunnel: [w747] -> w739
          stop <- "Next2" stop-if-true
          n375 = Wait Until Next ms Multiple(millisecond multiple=u32 100) -> ()  [unwired: 1 out]
        }
        n376 = property on="Video Camera" class="Ring (strict)"(error in=w739) -> (error out=w738:errorcluster, "RingText.Text"=→"Camera":string)  [unwired: 1 in, 1 out]
        n377 = call <vilib>:"Add State(s) to Queue__jki_lib_state_machine.vi"("State(s) in (\"\")"=w745) -> ("States Out"=w744:string)  [unwired: 14 in]
      }
    }
  }
  n378 = case shown="True" w4 {
    frame False {
    }
    frame True {
      n379 = local read "TestDefinition"() -> (w750:T4)
      n380 = Unbundle By Name(w750) -> ("Temperature Log Period(ms)"=w751:i64)
      n381 = while {
        tunnel: w751 -> [w765]
        stop <- w766 continue-if-true
        # "Display Trigger Value of  Temperatures"
        n382 = local read "TVC_Temperatures"() -> (w762:waveform(dbl)[])
        n383 = Wait Until Next ms Multiple(millisecond multiple=w765) -> ()  [unwired: 1 out]
        n384 = local read "ControlChannel"() -> (w760:u16)
        n385 = local read "Master Logging"() -> (w766:bool)
        n386 = Index Array(array=w762, index=w760) -> (element=w763:waveform(dbl))
        n387 = Unbundle By Name(w763) -> ("Y"=w764:dbl[])
        n388 = Index Array(array=w764) -> (element=→"Trigger Point Reading":dbl)  [unwired: 1 in]
      }
      n389 = local read "TopFolderPrefix"() -> (w754:string)
      n390 = local read "TopFolderPath"() -> (w755:path)
      n391 = Concatenate Strings(w754, "_Temp.xlsx") -> (w759:string)
      n392 = Build Path(base path=w755, name or relative path=w759) -> (appended path=w758:path)
      n393 = while {
        tunnel: w758 -> [w778]
        tunnel: w751 -> [w773]
        i -> [w771]
        stop <- w777 stop-if-true
        # "write Temperature log & graph\nwrite log file, buffer to memory\nflush on exit or every 100 readings"
        n394 = local read "Master Logging"() -> (w776:bool)
        n395 = Wait Until Next ms Multiple(millisecond multiple=w773) -> ()  [unwired: 1 out]
        n396 = local read "TLUP_Temperatures"() -> (w774:waveform(dbl)[])
        n397 = local read "TVC_Temperatures"() -> (w775:waveform(dbl)[])
        n398 = Quotient & Remainder(x=w771, y=100) -> (x-y*floor(x/y)=w769:i32)  [unwired: 1 out]
        n399 = Not(x=w776) -> (.not. x?=w777:bool)
        n400 = Equal To 0?(x=w769) -> (x = 0?=w768:bool)
        n401 = Or(x=w777, y=w768) -> (x .or. y?=w772:bool)
        n402 = Merge Signals(w775, w774) -> (w767:dynamicdata)
        "Temperatures" <- w767
        n403 = call "Write Master Temperature"("Signals"=w767, "Flush? (T)"=w772, "Filename"=w778) -> ()  [unwired: 14 in, 3 out]
      }
      n404 = Unbundle By Name(w750) -> ("PSU  Log Period (ms)"=w749:i64)
      n405 = Concatenate Strings(w754, "_PSU.xlsx") -> (w757:string)
      n406 = Build Path(base path=w755, name or relative path=w757) -> (appended path=w756:path)
      n407 = while {
        tunnel: w756 -> [w789]
        tunnel: w749 -> [w787]
        i -> [w781]
        stop <- w782 stop-if-true
        # "write Board PSU log\nwrite log file, buffer to memory\nflush on exit or every 100 readings"
        n408 = Wait Until Next ms Multiple(millisecond multiple=w787) -> ()  [unwired: 1 out]
        n409 = local read "Master Logging"() -> (w788:bool)
        n410 = local read "Heater Monitor"() -> (w786:waveform(dbl)[])
        n411 = local read "PSU_Monitor"() -> (w790:waveform(dbl)[])
        n412 = Quotient & Remainder(x=w781, y=1000) -> (x-y*floor(x/y)=w784:i32)  [unwired: 1 out]
        n413 = Not(x=w788) -> (.not. x?=w782:bool)
        n414 = Equal To 0?(x=w784) -> (x = 0?=w785:bool)
        n415 = Merge Signals(w786, w790) -> (w779:dynamicdata)
        "Current/Voltage" <- w779
        n416 = Or(x=w782, y=w785) -> (x .or. y?=w780:bool)
        n417 = call "Write Master PSU Log"("Signals"=w779, "Flush? (T)"=w780, "Filename"=w789) -> ()  [unwired: 14 in, 3 out]
      }
    }
  }
